vi "transfer char run_subvi_7_25_12b_JW.vi"(0 "VISA session":refnum<visa-resource-name>="GPIB0::17::INSTR", 5 "Var1 sweep settings":T4={"start"=40.0, "stop"=-40.0, "step (linear only)"=-1.0, "sweep spacing (linear: 0)"=0, "sweep mode"=FALSE, "compliance (V)"=100.0, "compliance (A)"=0.001} {"compliance (A)" format="%^.2e"; "compliance (V)" format="%.2f"; "sweep spacing (linear: 0)" items=["linear", "log 10", "log 25", "log 50"]; "step (linear only)" format="%.2f"; "stop" format="%.2f"; "start" format="%.2f"}, 7 "Var2 step settings":T3={"compliance (A)"=0.001, "compliance (V)"=100.0, "start"=-2.0, "total points"=2, "step"=-38.0} {"step" format="%.2f"; "start" format="%.2f"; "compliance (V)" format="%.2f"; "compliance (A)" format="%^.2e"}, 9 "integration time":u32(slide) scale=0.0..2.0, 11 "Input Path":path, 13 "Sample Properties:":T1 {"Date Created" format="%<%x>T"}) -> (1 "Trap Density-STS":dbl, 3 "Trap Density-VT":dbl, 4 "Mobility":dbl, 6 "graphic display":cluster{"trace":dbl[], "trace":dbl[]}(graph), 8 "On/Off Current":dbl, 10 "XY Graph":cluster{dbl[], "trace":dbl[]}[](graph), 12 "Vt":dbl, 14 "STS":dbl, 15 "error?":errorcluster)   [LabVIEW 2011]
uses:
  <vilib>/Utility/file.llb/Write To Spreadsheet File (DBL).vi
  <vilib>/Utility/file.llb/Read From Spreadsheet File (string).vi
  <vilib>/Utility/file.llb/Write To Spreadsheet File (string).vi
  <vilib>/Analysis/NI_AALPro.lvlib
panel:
  out "Test Array":string[][](array[string])
  out "Array":string[][](array[string])
  in  "Output Path":path
  in  "Temp (K)":dbl=0.001 format="%^.2e"
  in  "NumPts":dbl=5.0
  out "Numeric":dbl
  out "Max R":i32[](listbox)
  out "min r":dbl
  out "max r":dbl
  out "error? 2":errorcluster
  in  "MAXIMUM":ext format="%.2e"
  in  "MINIMUM":ext=-1e-05 format="%_2e"
  out "graphic display 2":cluster{"trace":dbl[], "trace":dbl[]}(graph)
  in  "Y1 axis":string="Id"
  in  "Y2 axis settings":T2 {"MAXIMUM" format="%.9f"; "MINIMUM" format="%.9f"}
  in  "wait time parameter":dbl=1.0
  in  "Value (Either V or A) 4":dbl
  in  "Value (Either V or A) 3":dbl
  in  "Value (Either V or A) 2":dbl
  in  "Value (V or A)":dbl
  in  "compliance (A)":dbl=0.001 format="%^.2e"
  in  "compliance (V)":dbl=100.0 format="%^.2e"
  in  "Iname":string="Is"
  in  "Vname":string="Vs"
  in  "Function":u16(ring)=4 items=["disabled", "Var1", "Var2", "Var1'", "Constant"]
  in  "Mode":u16(ring)=4 items=["V", "I", "VPulse", "IPulse", "Common"]
  in  "Iname 4":string="I4"
  in  "Vname 4":string="V4"
  in  "Function 4":u16(ring)=4 items=["disabled", "Var1", "Var2", "Var1'", "Constant"]
  in  "Mode 4":u16(ring) items=["V", "I", "VPulse", "IPulse", "Common"]
  in  "Iname 3":string="Ig"
  in  "Vname 3":string="Vg"
  in  "Function 3":u16(ring)=1 items=["disabled", "Var1", "Var2", "Var1'", "Constant"]
  in  "Mode 3":u16(ring) items=["V", "I", "VPulse", "IPulse", "Common"]
  in  "Iname 2":string="Id"
  in  "Vname 2":string="Vd"
  in  "Function 2":u16(ring)=2 items=["disabled", "Var1", "Var2", "Var1'", "Constant"]
  in  "Mode 2":u16(ring) items=["V", "I", "VPulse", "IPulse", "Common"]
  in  "reset":bool=TRUE
  # "SMU1"
  # "SMU2"
  # "SMU3"
  # "SMU4"
  # "Sample Properties:"
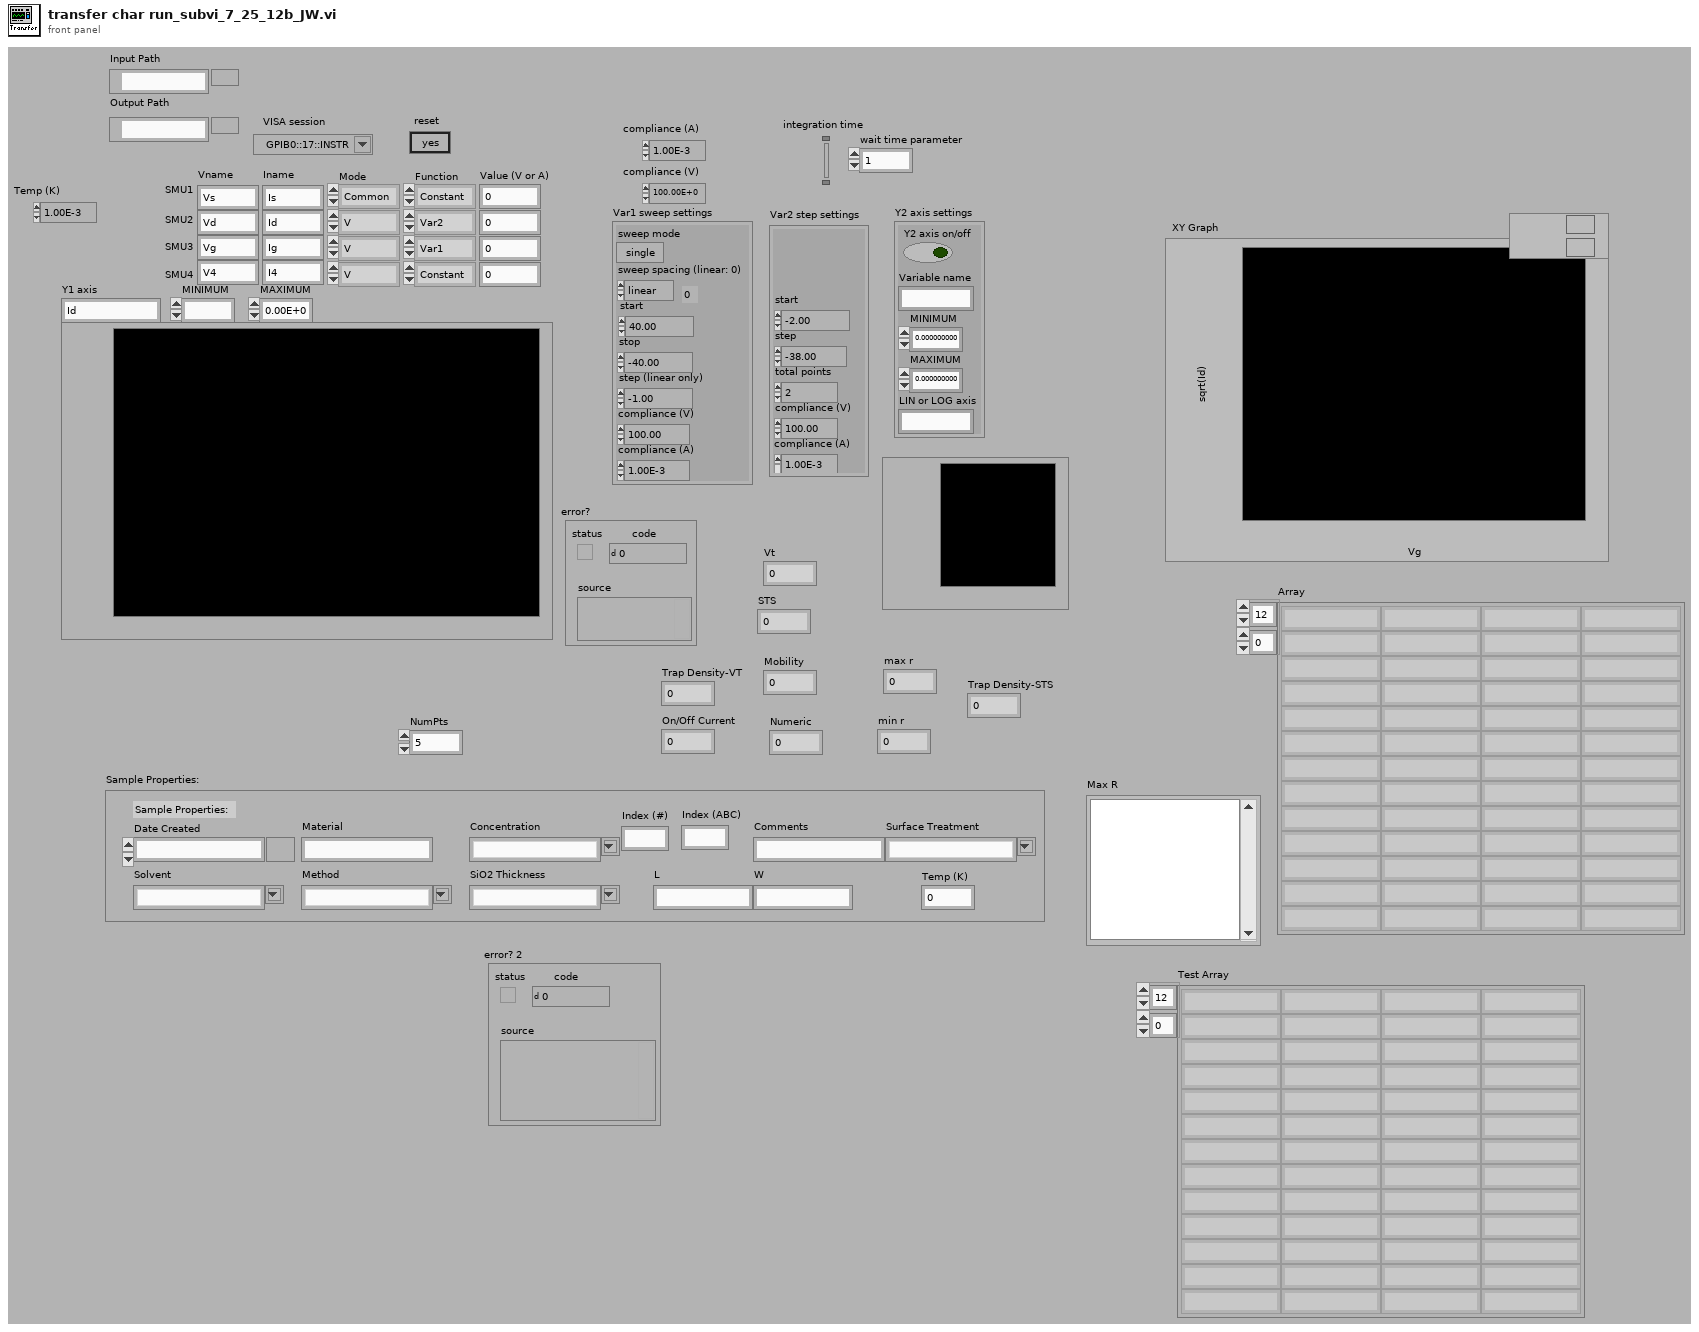
[diagram p1: front panel]
types:
  T1 = cluster{"Date Created":timestamp, "Material":string, "Solvent":string, "Concentration":string, "Method":string, "SiO2 Thickness":string, "Index (#)":string, "Index (ABC)":string, "L":string, "W":string, "Surface Treatment":string, "Comments":string, "Temp (K)":dbl}
  T2 = cluster{"Y2 axis on/off":bool, "MINIMUM":ext, "MAXIMUM":ext, "Variable name":string, "LIN or LOG axis":string}
  T3 = cluster{"compliance (A)":dbl, "compliance (V)":dbl, "start":dbl, "total points":u16, "step":dbl}
  T4 = cluster{"start":dbl, "stop":dbl, "step (linear only)":dbl, "sweep spacing (linear: 0)":u16, "sweep mode":bool, "compliance (V)":dbl, "compliance (A)":dbl}
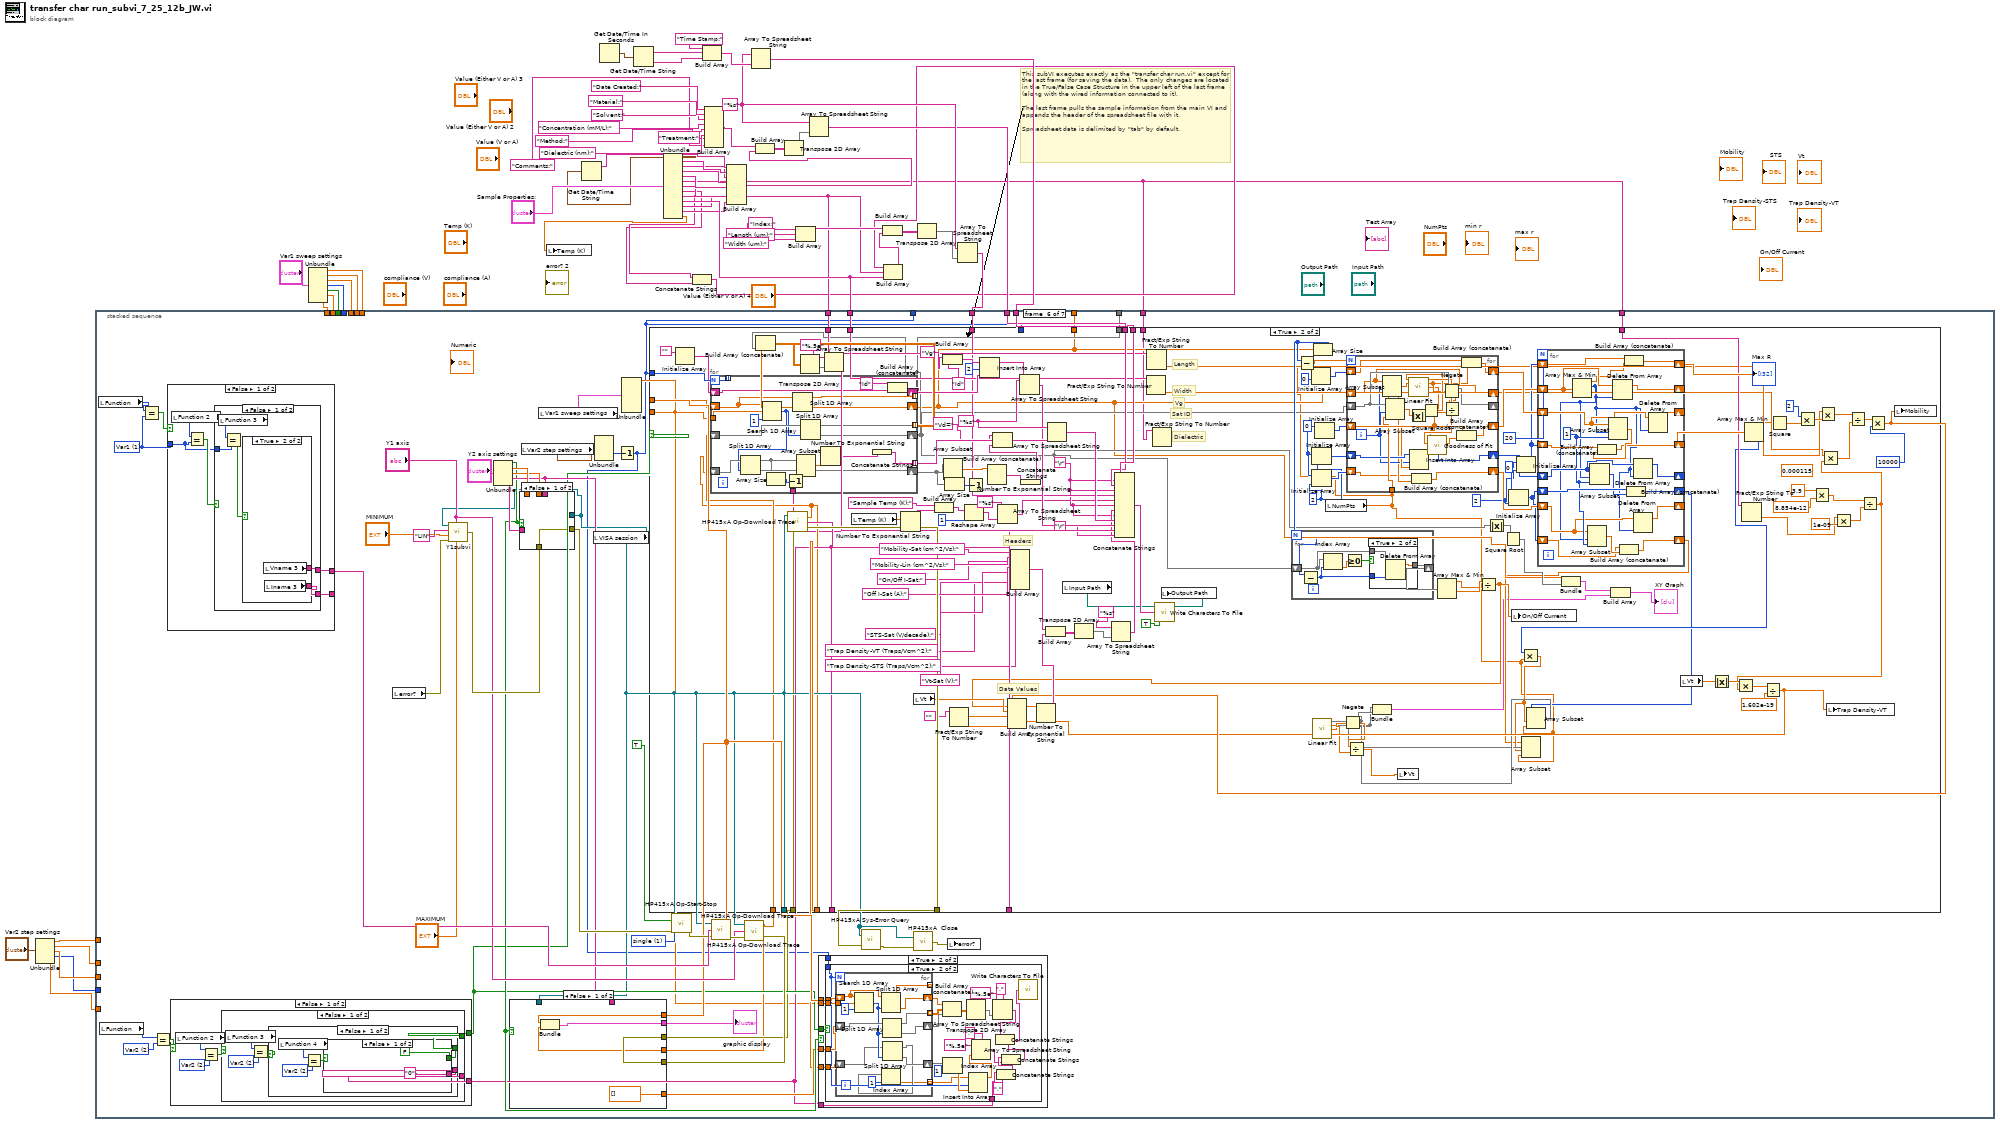
[diagram p0: block diagram]
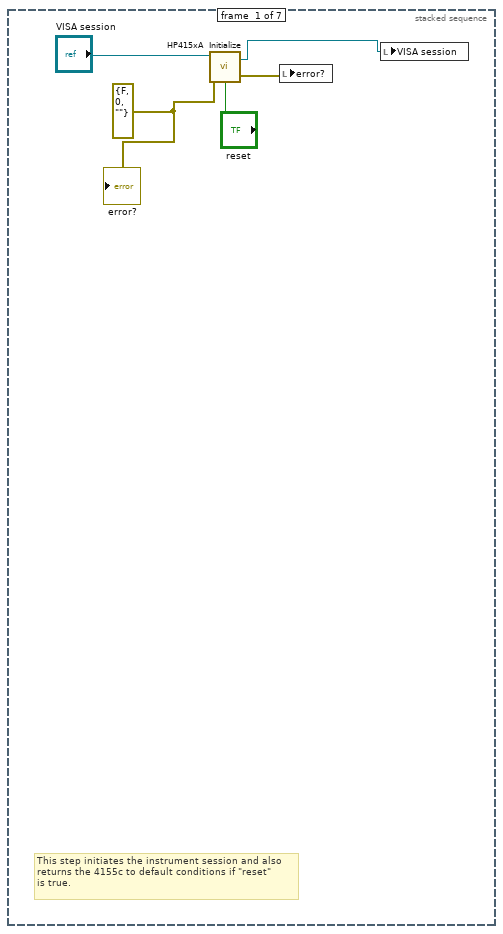
[diagram p2: hidden frame]
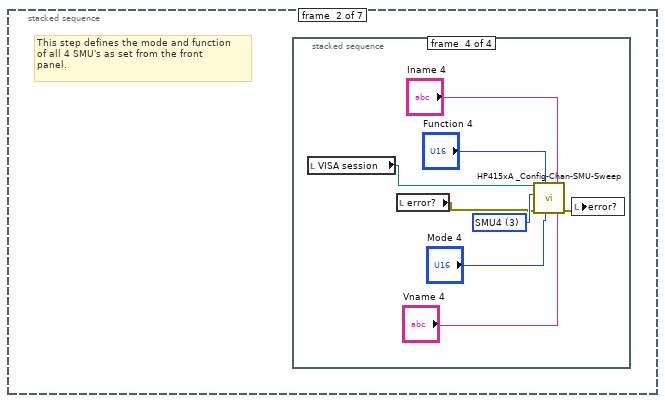
[diagram p3: hidden frame]
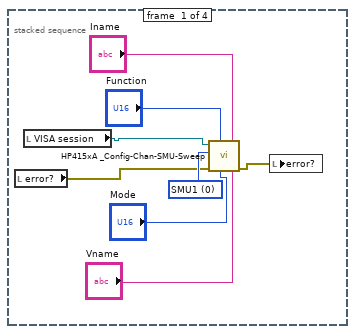
[diagram p4: hidden frame]
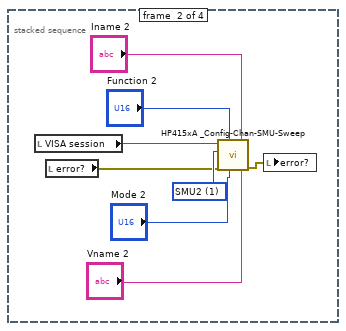
[diagram p5: hidden frame]
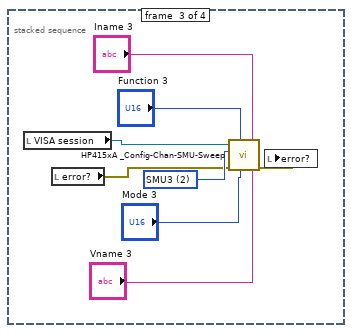
[diagram p6: hidden frame]
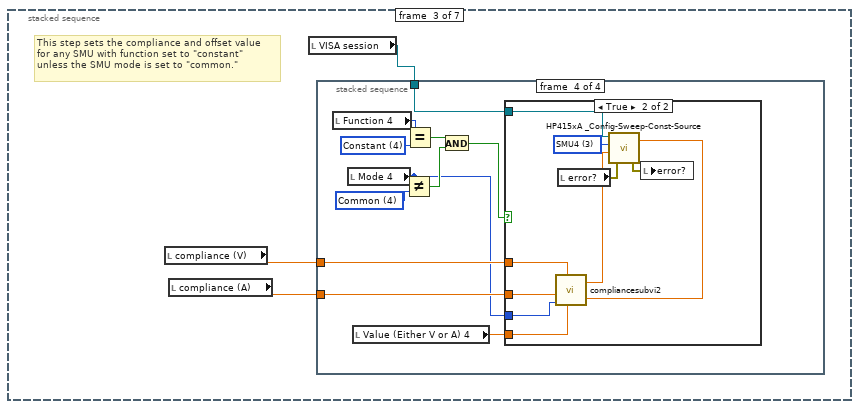
[diagram p7: hidden frame]
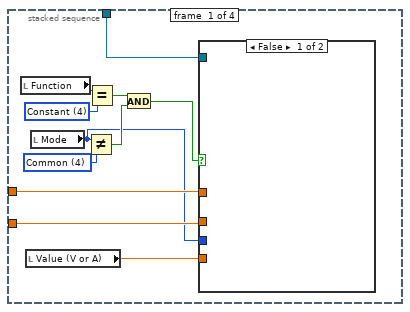
[diagram p8: hidden frame]
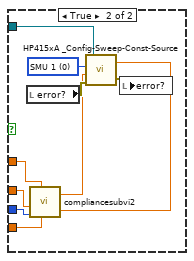
[diagram p9: hidden frame]
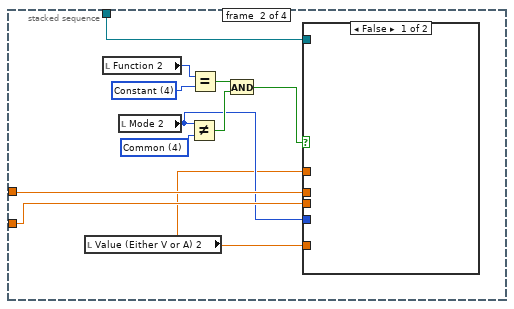
[diagram p10: hidden frame]
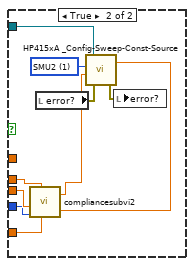
[diagram p11: hidden frame]
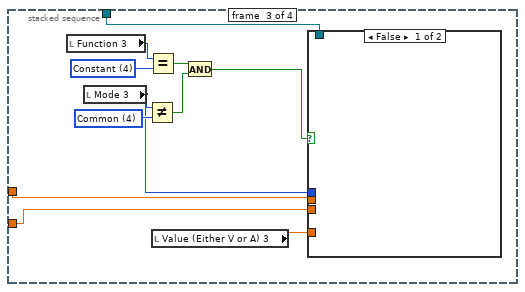
[diagram p12: hidden frame]
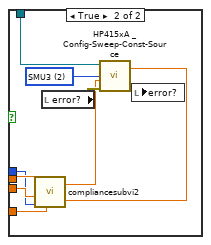
[diagram p13: hidden frame]
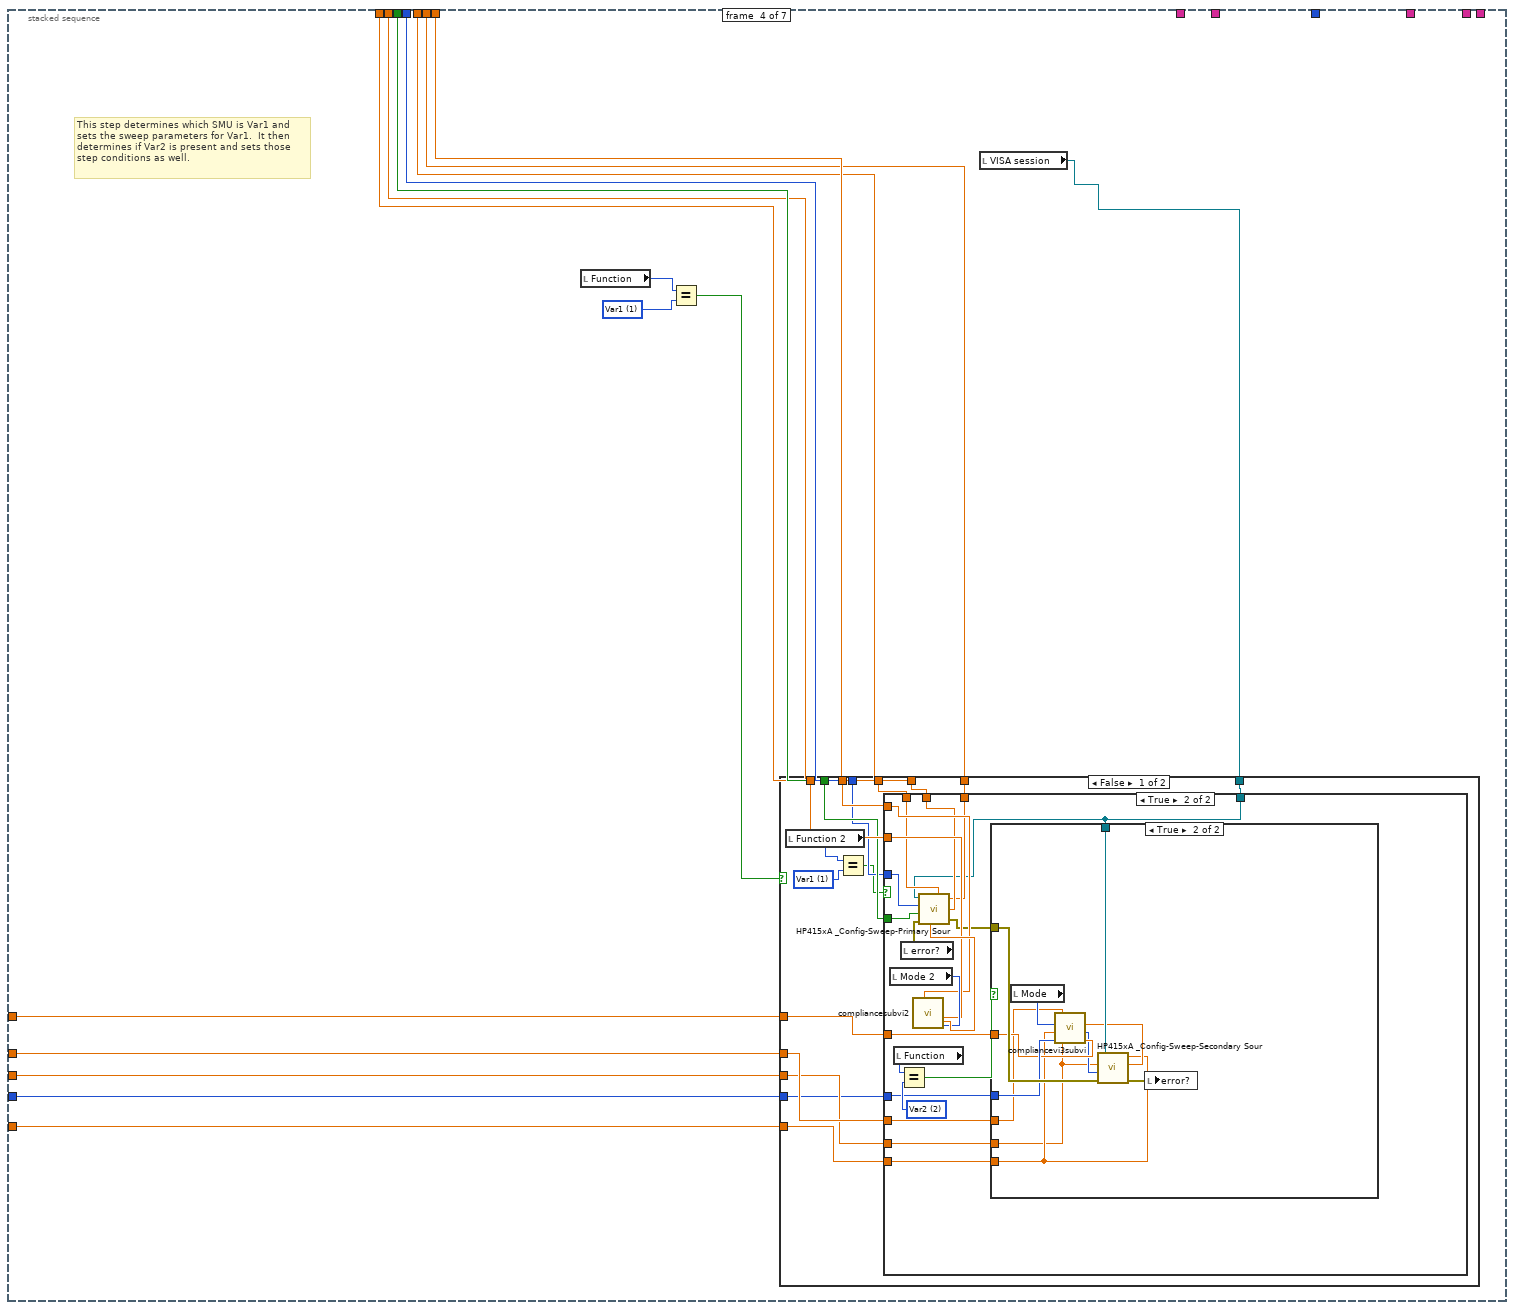
[diagram p15: hidden frame]
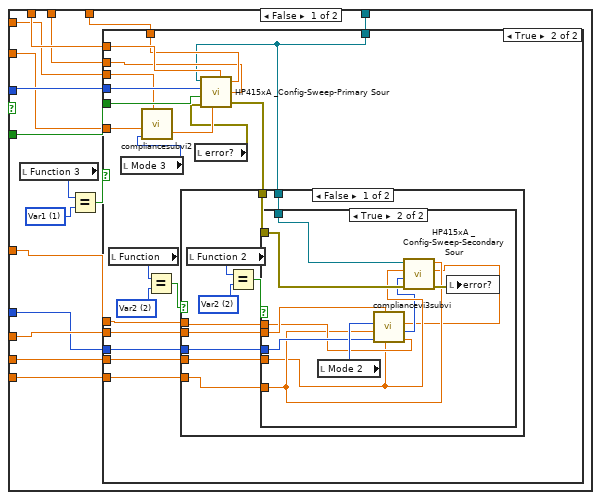
[diagram p16: hidden frame]
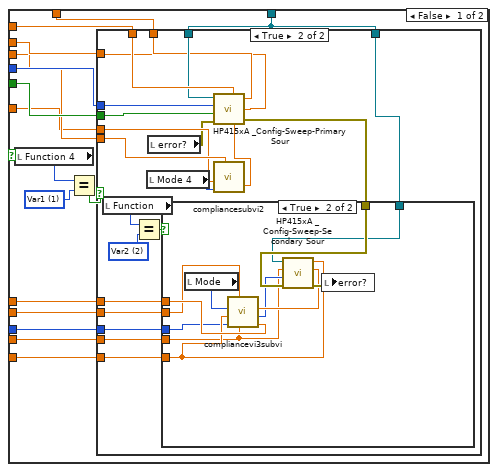
[diagram p17: hidden frame]
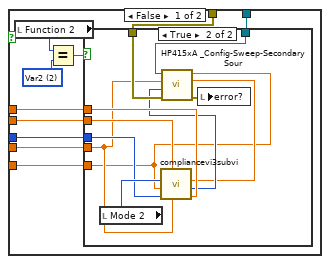
[diagram p19: hidden frame]
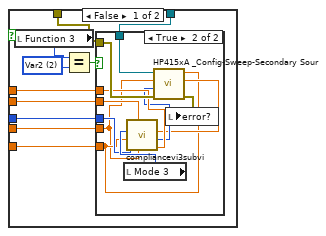
[diagram p20: hidden frame]
diagram:
  w31 = "%s"
  # "This subVI executes exactly as the \"transfer char run.vi\" except for the last frame (for saving the data).  The only changes are located in the True/False Case Structure in the upper left of the last frame (along with the wired information connected to it). \n\nThe last frame pulls the sample information from the main VI and appends the header of the spreadsheet file with it.\n\nSpreadsheet data is delimited by \"tab\" by default."
  n1 = Unbundle("Var2 step settings") -> ("compliance (A)"=w49:dbl, "compliance (V)"=w48:dbl, "start"=w47:dbl, "total points"=w46:u16, "step"=w45:dbl)
  n2 = Unbundle("Var1 sweep settings") -> ("start"=w57:dbl, "stop"=w56:dbl, "step (linear only)"=w55:dbl, "sweep spacing (linear: 0)"=w54:u16, "sweep mode"=w53:bool, "compliance (V)"=w52:dbl, "compliance (A)"=w51:dbl)
  n3 = Get Date/Time In Seconds() -> (seconds since 1Jan1904=w38:timestamp)
  n4 = Get Date/Time String(seconds (now)=w38) -> (date string=w37:string, time string=w36:string)  [unwired: 2 in]
  n5 = Unbundle("Sample Properties:") -> ("Date Created"=w16:timestamp, "Material"=w15:string, "Solvent"=w11:string, "Concentration"=w10:string, "Method"=w14:string, "SiO2 Thickness"=w1:string, "Index (#)"=w5:string, "Index (ABC)"=w4:string, "L"=w8:string, "W"=w9:string, "Surface Treatment"=w7:string, "Comments"=w6:string, "Temp (K)"=w2:dbl)
  n6 = local write "Temp (K)"(w2) -> ()
  n7 = Get Date/Time String(seconds (now)=w16) -> (date string=w43:string)  [unwired: 2 in, 1 out]
  n8 = Concatenate Strings(w5, w4) -> (w3:string)
  n9 = Build Array("Time Stamp:", w37, w36) -> (w35:string[])
  n10 = Build Array("Date Created:", "Material:", "Solvent:", "Concentration (mM/L):", "Method:", "Dielectric (nm):", "Treatment:", "Comments:") -> (w26:string[])
  n11 = Build Array(w43, w15, w11, w10, w14, w1, w7, w6) -> (w25:string[])
  n12 = Array To Spreadsheet String(array=w35, 3:w31) -> (spreadsheet string=w27:string)  [unwired: 1 in]
  n13 = Build Array(w26, w25) -> (w24:string[][])
  n14 = Transpose 2D Array(2D array=w24) -> (transposed array=w23:string[][])
  n15 = Build Array("Index:", "Length (um):", "Width (um):") -> (w22:string[])
  n16 = Array To Spreadsheet String(array=w23, 3:w31) -> (spreadsheet string=w30:string)  [unwired: 1 in]
  n17 = Build Array(w3, w8, w9) -> (w21:string[])
  n18 = Build Array(w22, w21) -> (w20:string[][])
  n19 = Transpose 2D Array(2D array=w20) -> (transposed array=w19:string[][])
  n20 = Array To Spreadsheet String(array=w19, 3:w31) -> (spreadsheet string=w18:string)  [unwired: 1 in]
  n21 = stacked-sequence {
    tunnel: w57 -> [_ _ _ w194 _ _ _]
    tunnel: w56 -> [_ _ _ w193 _ _ _]
    tunnel: w55 -> [_ _ _ w192 _ _ _]
    tunnel: w54 -> [_ _ _ w191 _ _ _]
    tunnel: w53 -> [_ _ _ w190 _ _ _]
    tunnel: w52 -> [_ _ _ w189 _ _ _]
    tunnel: w51 -> [_ _ _ w188 _ _ _]
    tunnel: w49 -> [_ _ _ w187 _ _ _]
    tunnel: w48 -> [_ _ _ w186 _ _ _]
    tunnel: w47 -> [_ _ _ w185 _ _ _]
    tunnel: w46 -> [_ _ _ w184 _ _ _]
    tunnel: w45 -> [_ _ _ w183 _ _ _]
    tunnel: w27 -> [_ _ _ _ _ w558 _]
    tunnel: w30 -> [_ _ _ _ _ w557 _]
    tunnel: w18 -> [_ _ _ _ _ w556 _]
    tunnel: [_ _ _ _ _ w555 _] -> _
    tunnel: [_ _ _ _ _ w554 _] -> _
    tunnel: [_ _ _ _ _ w551 _] -> _
    tunnel: w9 -> [_ _ _ _ _ w553 _]
    tunnel: w8 -> [_ _ _ _ _ w552 _]
    tunnel: w1 -> [_ _ _ _ _ w550 _]
    tunnel: w1 -> [_ _ _ _ _ w549 _]
    frame #0 {
      w62 = errorcluster {"status"=FALSE, "code"=0, "source"=""} ("error out")
      # "This step initiates the instrument session and also\nreturns the 4155c to default conditions if \"reset\"\nis true."
      n22 = call "HP415xA  Initialize.vi"("instrument descriptor"="VISA session", "reset"="reset", "error in (no error)"=w62) -> ("VISA session"=w59:refnum<visa-resource-name>, "error out"=w61:errorcluster)  [unwired: 2 in]
      n23 = local write "error?"(w61) -> ()
      n24 = local write "VISA session"(w59) -> ()
      "error?" <- w62
    }
    frame #1 {
      # "This step defines the mode and function\nof all 4 SMU's as set from the front\npanel."
      n25 = stacked-sequence {
        frame #0 {
          w71 = u32 0 items=["SMU1  ", "SMU2  ", "SMU3  ", "SMU4  ", "SMU5  ", "SMU6  "] ("unit to configure")
          n26 = local read "error?"() -> (w66:errorcluster)
          n27 = local read "VISA session"() -> (w64:refnum<visa-resource-name>)
          n28 = call "HP415xA _Config-Chan-SMU-Sweep.vi"("V name (max 6 chars)"="Vname", "I name (max 6 chars)"="Iname", "mode"="Mode", "function"="Function", "error in (no error)"=w66, "unit to configure"=w71, "VISA session"=w64) -> ("error out"=w65:errorcluster)  [unwired: 2 in]
          n29 = local write "error?"(w65) -> ()
        }
        frame #1 {
          w75 = u32 1 items=["SMU1  ", "SMU2  ", "SMU3  ", "SMU4  ", "SMU5  ", "SMU6  "] ("unit to configure")
          n30 = local read "VISA session"() -> (w72:refnum<visa-resource-name>)
          n31 = local read "error?"() -> (w73:errorcluster)
          n32 = call "HP415xA _Config-Chan-SMU-Sweep.vi"("V name (max 6 chars)"="Vname 2", "I name (max 6 chars)"="Iname 2", "mode"="Mode 2", "function"="Function 2", "error in (no error)"=w73, "unit to configure"=w75, "VISA session"=w72) -> ("error out"=w74:errorcluster)  [unwired: 2 in]
          n33 = local write "error?"(w74) -> ()
        }
        frame #2 {
          w83 = u32 2 items=["SMU1  ", "SMU2  ", "SMU3  ", "SMU4  ", "SMU5  ", "SMU6  "] ("unit to configure")
          n34 = local read "VISA session"() -> (w80:refnum<visa-resource-name>)
          n35 = local read "error?"() -> (w81:errorcluster)
          n36 = call "HP415xA _Config-Chan-SMU-Sweep.vi"("V name (max 6 chars)"="Vname 3", "I name (max 6 chars)"="Iname 3", "mode"="Mode 3", "function"="Function 3", "error in (no error)"=w81, "unit to configure"=w83, "VISA session"=w80) -> ("error out"=w82:errorcluster)  [unwired: 2 in]
          n37 = local write "error?"(w82) -> ()
        }
        frame #3 {
          w91 = u32 3 items=["SMU1  ", "SMU2  ", "SMU3  ", "SMU4  ", "SMU5  ", "SMU6  "] ("unit to configure")
          n38 = local read "VISA session"() -> (w88:refnum<visa-resource-name>)
          n39 = local read "error?"() -> (w90:errorcluster)
          n40 = call "HP415xA _Config-Chan-SMU-Sweep.vi"("V name (max 6 chars)"="Vname 4", "I name (max 6 chars)"="Iname 4", "mode"="Mode 4", "function"="Function 4", "error in (no error)"=w90, "unit to configure"=w91, "VISA session"=w88) -> ("error out"=w89:errorcluster)  [unwired: 2 in]
          n41 = local write "error?"(w89) -> ()
        }
      }
    }
    frame #2 {
      # "This step sets the compliance and offset value\nfor any SMU with function set to \"constant\"\nunless the SMU mode is set to \"common.\""
      n42 = local read "compliance (V)"() -> (w97:dbl)
      n43 = local read "compliance (A)"() -> (w98:dbl)
      n44 = local read "VISA session"() -> (w96:refnum<visa-resource-name>)
      n45 = stacked-sequence {
        tunnel: w96 -> [w107 w127 w146 w166]
        tunnel: w98 -> [w101 w123 w144 w164]
        tunnel: w97 -> [w100 w122 w143 w165]
        frame #0 {
          w105 = u16 4 items=["V", "I", "VPulse", "IPulse", "Common"] ("Mode")
          w109 = u16 4 items=["disabled", "Var1", "Var2", "Var1'", "Constant"] ("Function")
          n46 = local read "Function"() -> (w108:u16)
          n47 = local read "Value (V or A)"() -> (w102:dbl)
          n48 = local read "Mode"() -> (w99:u16)
          n49 = Not Equal?(x=w99, y=w105) -> (x != y?=w104:bool)
          n50 = Equal?(x=w108, y=w109) -> (x = y?=w106:bool)
          n51 = And(x=w106, y=w104) -> (x .and. y?=w103:bool)
          n52 = case shown="False" w103 {
            tunnel: w107 -> [_ w119]
            tunnel: w100 -> [_ w115]
            tunnel: w101 -> [_ w114]
            tunnel: w102 -> [_ w111]
            tunnel: w99 -> [_ w112]
            frame False {
            }
            frame True {
              w118 = u16 0 items=["SMU 1", "SMU2", "SMU3", "SMU4", "SMU5", "SMU6", "VSU1", "VSU2"] ("unit (SMU1:0)")
              n53 = local read "error?"() -> (w117:errorcluster)
              n54 = call "compliancesubvi2.vi"("Value1"=w111, "compliance (V)"=w115, "Mode"=w112, "compliance (A)"=w114) -> ("compliance"=w113:dbl, "constant"=w110:dbl)  [unwired: 2 in]
              n55 = call "HP415xA _Config-Sweep-Const-Source.vi"("compliance (SMUs only)"=w113, "error in (no error)"=w117, "source (V or A)"=w110, "unit (SMU1:0)"=w118, "VISA session"=w119) -> ("error out"=w116:errorcluster)
              n56 = local write "error?"(w116) -> ()
            }
          }
        }
        frame #1 {
          w124 = u16 4 items=["V", "I", "VPulse", "IPulse", "Common"] ("Mode 2")
          w125 = u16 4 items=["disabled", "Var1", "Var2", "Var1'", "Constant"] ("Function 2")
          n57 = local read "Value (Either V or A) 2"() -> (w120:dbl)
          n58 = local read "Function 2"() -> (w126:u16)
          n59 = local read "Mode 2"() -> (w121:u16)
          n60 = Not Equal?(x=w121, y=w124) -> (x != y?=w129:bool)
          n61 = Equal?(x=w126, y=w125) -> (x = y?=w130:bool)
          n62 = And(x=w130, y=w129) -> (x .and. y?=w128:bool)
          n63 = case shown="False" w128 {
            tunnel: w127 -> [_ w140]
            tunnel: w122 -> [_ w138]
            tunnel: w123 -> [_ w137]
            tunnel: w120 -> [_ _]
            tunnel: w121 -> [_ w133]
            tunnel: w120 -> [_ w132]
            frame False {
            }
            frame True {
              w139 = u16 1 items=["SMU 1", "SMU2", "SMU3", "SMU4", "SMU5", "SMU6", "VSU1", "VSU2"] ("unit (SMU1:0)")
              n64 = call "compliancesubvi2.vi"("Value1"=w132, "compliance (V)"=w138, "Mode"=w133, "compliance (A)"=w137) -> ("compliance"=w136:dbl, "constant"=w131:dbl)  [unwired: 2 in]
              n65 = local read "error?"() -> (w135:errorcluster)
              n66 = call "HP415xA _Config-Sweep-Const-Source.vi"("compliance (SMUs only)"=w136, "error in (no error)"=w135, "source (V or A)"=w131, "unit (SMU1:0)"=w139, "VISA session"=w140) -> ("error out"=w134:errorcluster)
              n67 = local write "error?"(w134) -> ()
            }
          }
        }
        frame #2 {
          w148 = u16 4 items=["V", "I", "VPulse", "IPulse", "Common"] ("Mode 2")
          w149 = u16 4 items=["disabled", "Var1", "Var2", "Var1'", "Constant"] ("Function 2")
          n68 = local read "Function 3"() -> (w147:u16)
          n69 = local read "Mode 3"() -> (w142:u16)
          n70 = Not Equal?(x=w142, y=w148) -> (x != y?=w150:bool)
          n71 = Equal?(x=w147, y=w149) -> (x = y?=w151:bool)
          n72 = local read "Value (Either V or A) 3"() -> (w145:dbl)
          n73 = And(x=w151, y=w150) -> (x .and. y?=w141:bool)
          n74 = case shown="False" w141 {
            tunnel: w146 -> [_ w159]
            tunnel: w145 -> [_ w153]
            tunnel: w144 -> [_ w156]
            tunnel: w143 -> [_ w155]
            tunnel: w142 -> [_ w154]
            frame False {
            }
            frame True {
              w158 = u16 2 items=["SMU 1", "SMU2", "SMU3", "SMU4", "SMU5", "SMU6", "VSU1", "VSU2"] ("unit (SMU1:0)")
              n75 = call "compliancesubvi2.vi"("Value1"=w153, "compliance (V)"=w155, "Mode"=w154, "compliance (A)"=w156) -> ("compliance"=w157:dbl, "constant"=w152:dbl)  [unwired: 2 in]
              n76 = local read "error?"() -> (w161:errorcluster)
              n77 = call "HP415xA _Config-Sweep-Const-Source.vi"("compliance (SMUs only)"=w157, "error in (no error)"=w161, "source (V or A)"=w152, "unit (SMU1:0)"=w158, "VISA session"=w159) -> ("error out"=w160:errorcluster)
              n78 = local write "error?"(w160) -> ()
            }
          }
        }
        frame #3 {
          w168 = u16 4 items=["V", "I", "VPulse", "IPulse", "Common"] ("Mode 4")
          w169 = u16 4 items=["disabled", "Var1", "Var2", "Var1'", "Constant"] ("Function 4")
          n79 = local read "Function 4"() -> (w170:u16)
          n80 = local read "Mode 4"() -> (w163:u16)
          n81 = local read "Value (Either V or A) 4"() -> (w162:dbl)
          n82 = Not Equal?(x=w163, y=w168) -> (x != y?=w171:bool)
          n83 = Equal?(x=w170, y=w169) -> (x = y?=w172:bool)
          n84 = And(x=w172, y=w171) -> (x .and. y?=w167:bool)
          n85 = case shown="True" w167 {
            tunnel: w166 -> [_ w181]
            tunnel: w165 -> [_ w177]
            tunnel: w164 -> [_ w178]
            tunnel: w163 -> [_ w176]
            tunnel: w162 -> [_ w175]
            frame False {
            }
            frame True {
              w182 = u16 3 items=["SMU 1", "SMU2", "SMU3", "SMU4", "SMU5", "SMU6", "VSU1", "VSU2"] ("unit (SMU1:0)")
              n86 = call "compliancesubvi2.vi"("Value1"=w175, "compliance (V)"=w177, "Mode"=w176, "compliance (A)"=w178) -> ("compliance"=w174:dbl, "constant"=w173:dbl)  [unwired: 2 in]
              n87 = local read "error?"() -> (w180:errorcluster)
              n88 = call "HP415xA _Config-Sweep-Const-Source.vi"("compliance (SMUs only)"=w174, "error in (no error)"=w180, "source (V or A)"=w173, "unit (SMU1:0)"=w182, "VISA session"=w181) -> ("error out"=w179:errorcluster)
              n89 = local write "error?"(w179) -> ()
            }
          }
        }
      }
    }
    frame #3 {
      w198 = u16 1 items=["disabled", "Var1", "Var2", "Var1'", "Constant"] ("Function")
      # "This step determines which SMU is Var1 and\nsets the sweep parameters for Var1.  It then\ndetermines if Var2 is present and sets those\nstep conditions as well."
      n90 = local read "Function"() -> (w197:u16)
      n91 = Equal?(x=w197, y=w198) -> (x = y?=w196:bool)
      n92 = local read "VISA session"() -> (w195:refnum<visa-resource-name>)
      n93 = case shown="False" w196 {
        tunnel: w189 -> [w211 w487]
        tunnel: w188 -> [w212 w486]
        tunnel: w191 -> [w209 w485]
        tunnel: w190 -> [w210 w484]
        tunnel: w192 -> [w206 w483]
        tunnel: w193 -> [w205 w482]
        tunnel: w194 -> [w207 w481]
        tunnel: w195 -> [w208 w470]
        tunnel: w187 -> [w203 w476]
        tunnel: w186 -> [w202 w475]
        tunnel: w185 -> [w201 w474]
        tunnel: w184 -> [w200 w473]
        tunnel: w183 -> [w199 w472]
        frame False {
          w214 = u16 1 items=["disabled", "Var1", "Var2", "Var1'", "Constant"] ("Function")
          n94 = local read "Function 2"() -> (w213:u16)
          n95 = Equal?(x=w213, y=w214) -> (x = y?=w204:bool)
          n96 = case shown="True" w204 {
            tunnel: w212 -> [w220 w413]
            tunnel: w211 -> [w221 w412]
            tunnel: w210 -> [w222 w411]
            tunnel: w209 -> [w223 w410]
            tunnel: w208 -> [w227 w399]
            tunnel: w207 -> [w226 w409]
            tunnel: w206 -> [w224 w408]
            tunnel: w205 -> [w225 w407]
            tunnel: w203 -> [w219 w402]
            tunnel: w202 -> [w218 w401]
            tunnel: w201 -> [w216 w400]
            tunnel: w200 -> [w217 w397]
            tunnel: w199 -> [w215 w396]
            frame False {
              w230 = u16 1 items=["disabled", "Var1", "Var2", "Var1'", "Constant"] ("Function")
              n97 = local read "Function 3"() -> (w229:u16)
              n98 = Equal?(x=w229, y=w230) -> (x = y?=w228:bool)
              n99 = case shown="True" w228 {
                tunnel: w227 -> [w231 w324]
                tunnel: w226 -> [w243 w341]
                tunnel: w225 -> [w240 w340]
                tunnel: w224 -> [w239 w339]
                tunnel: w223 -> [w242 w338]
                tunnel: w222 -> [w241 w337]
                tunnel: w221 -> [w238 w336]
                tunnel: w220 -> [w237 w335]
                tunnel: w219 -> [w236 w328]
                tunnel: w218 -> [w235 w327]
                tunnel: w217 -> [w234 w326]
                tunnel: w216 -> [w233 w323]
                tunnel: w215 -> [w232 w322]
                frame False {
                  w246 = u16 1 items=["disabled", "Var1", "Var2", "Var1'", "Constant"] ("Function")
                  n100 = local read "Function 4"() -> (w245:u16)
                  n101 = Equal?(x=w245, y=w246) -> (x = y?=w244:bool)
                  n102 = case shown="True" w244 {
                    tunnel: w243 -> [_ w265]
                    tunnel: w231 -> [_ w264]
                    tunnel: w242 -> [_ w263]
                    tunnel: w241 -> [_ w262]
                    tunnel: w240 -> [_ w261]
                    tunnel: w239 -> [_ w260]
                    tunnel: w238 -> [_ w259]
                    tunnel: w237 -> [_ w258]
                    tunnel: w236 -> [_ w253]
                    tunnel: w235 -> [_ w252]
                    tunnel: w234 -> [_ w251]
                    tunnel: w233 -> [_ w250]
                    tunnel: w232 -> [_ w249]
                    tunnel: w231 -> [_ w247]
                    frame False {
                    }
                    frame True {
                      w256 = u16 2 items=["disabled", "Var1", "Var2", "Var1'", "Constant"] ("Function")
                      n103 = local read "Function"() -> (w255:u16)
                      n104 = Equal?(x=w255, y=w256) -> (x = y?=w254:bool)
                      n105 = local read "Mode 4"() -> (w267:u16)
                      n106 = local read "error?"() -> (w257:errorcluster)
                      n107 = call "compliancesubvi2.vi"("compliance (V)"=w259, "Mode"=w267, "compliance (A)"=w258) -> ("compliance"=w266:dbl)  [unwired: 3 in, 1 out]
                      n108 = call "HP415xA _Config-Sweep-Primary Sour.vi"("step (linear only)"=w260, "stop"=w261, "start"=w265, "compliance"=w266, "error in (no error)"=w257, "sweep mode"=w262, "sweep spacing (linear: 0)"=w263, "VISA session"=w264) -> ("error out"=w248:errorcluster)  [unwired: 2 in]
                      n109 = case shown="True" w254 {
                        tunnel: w253 -> [w274 w317]
                        tunnel: w252 -> [w273 w312]
                        tunnel: w251 -> [w272 w311]
                        tunnel: w250 -> [w271 w313]
                        tunnel: w249 -> [w270 w316]
                        tunnel: w248 -> [w269 w319]
                        tunnel: w247 -> [w268 w318]
                        frame False {
                          w277 = u16 2 items=["disabled", "Var1", "Var2", "Var1'", "Constant"] ("Function")
                          n110 = local read "Function 2"() -> (w276:u16)
                          n111 = Equal?(x=w276, y=w277) -> (x = y?=w275:bool)
                          n112 = case shown="True" w275 {
                            tunnel: w274 -> [w285 w305]
                            tunnel: w273 -> [w284 w306]
                            tunnel: w272 -> [w283 w304]
                            tunnel: w271 -> [w282 w302]
                            tunnel: w270 -> [w281 w300]
                            tunnel: w269 -> [w280 w310]
                            tunnel: w268 -> [w278 w309]
                            frame False {
                              w287 = u16 2 items=["disabled", "Var1", "Var2", "Var1'", "Constant"] ("Function")
                              n113 = local read "Function 3"() -> (w279:u16)
                              n114 = Equal?(x=w279, y=w287) -> (x = y?=w286:bool)
                              n115 = case shown="True" w286 {
                                tunnel: w285 -> [_ w293]
                                tunnel: w284 -> [_ w294]
                                tunnel: w283 -> [_ w295]
                                tunnel: w282 -> [_ w289]
                                tunnel: w281 -> [_ w290]
                                tunnel: w280 -> [w288 w299]
                                tunnel: w278 -> [_ w298]
                                frame False {
                                n116 = local write "error?"(w288) -> ()
                                }
                                frame True {
                                n117 = local read "Mode 3"() -> (w297:u16)
                                n118 = call "compliancevi3subvi.vi"("compliance (A)"=w293, "start"=w289, "compliance (V)"=w294, "total points"=w295, "step"=w290, "Mode"=w297) -> ("total points 2"=w292:u16, "compliance"=w291:dbl)  [unwired: 1 in, 1 out]
                                n119 = call "HP415xA _Config-Sweep-Secondary Sour.vi"("compliance"=w291, "step"=w290, "error in (no error)"=w299, "total points"=w292, "start"=w289, "VISA session"=w298) -> ("error out"=w296:errorcluster)  [unwired: 1 in]
                                n120 = local write "error?"(w296) -> ()
                                }
                              }
                            }
                            frame True {
                              n121 = local read "Mode 2"() -> (w308:u16)
                              n122 = call "compliancevi3subvi.vi"("compliance (A)"=w305, "start"=w302, "compliance (V)"=w306, "total points"=w304, "step"=w300, "Mode"=w308) -> ("total points 2"=w303:u16, "compliance"=w301:dbl)  [unwired: 1 in, 1 out]
                              n123 = call "HP415xA _Config-Sweep-Secondary Sour.vi"("compliance"=w301, "step"=w300, "error in (no error)"=w310, "total points"=w303, "start"=w302, "VISA session"=w309) -> ("error out"=w307:errorcluster)  [unwired: 1 in]
                              n124 = local write "error?"(w307) -> ()
                            }
                          }
                        }
                        frame True {
                          n125 = local read "Mode"() -> (w321:u16)
                          n126 = call "compliancevi3subvi.vi"("compliance (A)"=w317, "start"=w313, "compliance (V)"=w312, "total points"=w311, "step"=w316, "Mode"=w321) -> ("total points 2"=w314:u16, "compliance"=w315:dbl)  [unwired: 1 in, 1 out]
                          n127 = call "HP415xA _Config-Sweep-Secondary Sour.vi"("compliance"=w315, "step"=w316, "error in (no error)"=w319, "total points"=w314, "start"=w313, "VISA session"=w318) -> ("error out"=w320:errorcluster)  [unwired: 1 in]
                          n128 = local write "error?"(w320) -> ()
                        }
                      }
                    }
                  }
                }
                frame True {
                  w331 = u16 2 items=["disabled", "Var1", "Var2", "Var1'", "Constant"] ("Function")
                  n129 = local read "Function"() -> (w330:u16)
                  n130 = local read "Mode 3"() -> (w333:u16)
                  n131 = call "compliancesubvi2.vi"("compliance (V)"=w336, "Mode"=w333, "compliance (A)"=w335) -> ("compliance"=w334:dbl)  [unwired: 3 in, 1 out]
                  n132 = Equal?(x=w330, y=w331) -> (x = y?=w329:bool)
                  n133 = local read "error?"() -> (w332:errorcluster)
                  n134 = call "HP415xA _Config-Sweep-Primary Sour.vi"("step (linear only)"=w339, "stop"=w340, "start"=w341, "compliance"=w334, "error in (no error)"=w332, "sweep mode"=w337, "sweep spacing (linear: 0)"=w338, "VISA session"=w324) -> ("error out"=w325:errorcluster)  [unwired: 2 in]
                  n135 = case shown="False" w329 {
                    tunnel: w328 -> [w346 w391]
                    tunnel: w327 -> [w345 w390]
                    tunnel: w326 -> [w343 w389]
                    tunnel: w325 -> [w348 w394]
                    tunnel: w324 -> [w347 w393]
                    tunnel: w323 -> [w342 w386]
                    tunnel: w322 -> [w344 w385]
                    frame False {
                      w351 = u16 2 items=["disabled", "Var1", "Var2", "Var1'", "Constant"] ("Function")
                      n136 = local read "Function 2"() -> (w350:u16)
                      n137 = Equal?(x=w350, y=w351) -> (x = y?=w349:bool)
                      n138 = case shown="True" w349 {
                        tunnel: w348 -> [w358 w383]
                        tunnel: w347 -> [w357 w382]
                        tunnel: w346 -> [w356 w378]
                        tunnel: w345 -> [w355 w379]
                        tunnel: w344 -> [w352 w377]
                        tunnel: w343 -> [w354 w380]
                        tunnel: w342 -> [w353 w376]
                        frame False {
                          w361 = u16 2 items=["disabled", "Var1", "Var2", "Var1'", "Constant"] ("Function")
                          n139 = local read "Function 4"() -> (w360:u16)
                          n140 = Equal?(x=w360, y=w361) -> (x = y?=w359:bool)
                          n141 = case shown="True" w359 {
                            tunnel: w358 -> [w362 w371]
                            tunnel: w357 -> [_ w372]
                            tunnel: w356 -> [_ w368]
                            tunnel: w355 -> [_ w369]
                            tunnel: w354 -> [_ w367]
                            tunnel: w353 -> [_ w364]
                            tunnel: w352 -> [_ w363]
                            frame False {
                              n142 = local write "error?"(w362) -> ()
                            }
                            frame True {
                              n143 = local read "Mode 4"() -> (w373:u16)
                              n144 = call "compliancevi3subvi.vi"("compliance (A)"=w368, "start"=w364, "compliance (V)"=w369, "total points"=w367, "step"=w363, "Mode"=w373) -> ("total points 2"=w366:u16, "compliance"=w365:dbl)  [unwired: 1 in, 1 out]
                              n145 = call "HP415xA _Config-Sweep-Secondary Sour.vi"("compliance"=w365, "step"=w363, "error in (no error)"=w371, "total points"=w366, "start"=w364, "VISA session"=w372) -> ("error out"=w370:errorcluster)  [unwired: 1 in]
                              n146 = local write "error?"(w370) -> ()
                            }
                          }
                        }
                        frame True {
                          n147 = local read "Mode 2"() -> (w384:u16)
                          n148 = call "compliancevi3subvi.vi"("compliance (A)"=w378, "start"=w376, "compliance (V)"=w379, "total points"=w380, "step"=w377, "Mode"=w384) -> ("total points 2"=w375:u16, "compliance"=w374:dbl)  [unwired: 1 in, 1 out]
                          n149 = call "HP415xA _Config-Sweep-Secondary Sour.vi"("compliance"=w374, "step"=w377, "error in (no error)"=w383, "total points"=w375, "start"=w376, "VISA session"=w382) -> ("error out"=w381:errorcluster)  [unwired: 1 in]
                          n150 = local write "error?"(w381) -> ()
                        }
                      }
                    }
                    frame True {
                      n151 = local read "Mode"() -> (w395:u16)
                      n152 = call "compliancevi3subvi.vi"("compliance (A)"=w391, "start"=w386, "compliance (V)"=w390, "total points"=w389, "step"=w385, "Mode"=w395) -> ("total points 2"=w388:u16, "compliance"=w387:dbl)  [unwired: 1 in, 1 out]
                      n153 = call "HP415xA _Config-Sweep-Secondary Sour.vi"("compliance"=w387, "step"=w385, "error in (no error)"=w394, "total points"=w388, "start"=w386, "VISA session"=w393) -> ("error out"=w392:errorcluster)  [unwired: 1 in]
                      n154 = local write "error?"(w392) -> ()
                    }
                  }
                }
              }
            }
            frame True {
              w405 = u16 2 items=["disabled", "Var1", "Var2", "Var1'", "Constant"] ("Function")
              n155 = local read "Mode 2"() -> (w414:u16)
              n156 = local read "Function"() -> (w404:u16)
              n157 = Equal?(x=w404, y=w405) -> (x = y?=w403:bool)
              n158 = local read "error?"() -> (w406:errorcluster)
              n159 = call "compliancesubvi2.vi"("compliance (V)"=w412, "Mode"=w414, "compliance (A)"=w413) -> ("compliance"=w415:dbl)  [unwired: 3 in, 1 out]
              n160 = call "HP415xA _Config-Sweep-Primary Sour.vi"("step (linear only)"=w408, "stop"=w407, "start"=w409, "compliance"=w415, "error in (no error)"=w406, "sweep mode"=w411, "sweep spacing (linear: 0)"=w410, "VISA session"=w399) -> ("error out"=w398:errorcluster)  [unwired: 2 in]
              n161 = case shown="True" w403 {
                tunnel: w402 -> [w421 w464]
                tunnel: w401 -> [w420 w463]
                tunnel: w400 -> [w418 w459]
                tunnel: w399 -> [w423 w469]
                tunnel: w398 -> [w417 w468]
                tunnel: w397 -> [w419 w465]
                tunnel: w396 -> [w416 w461]
                frame False {
                  w425 = u16 2 items=["disabled", "Var1", "Var2", "Var1'", "Constant"] ("Function")
                  n162 = local read "Function 3"() -> (w424:u16)
                  n163 = Equal?(x=w424, y=w425) -> (x = y?=w422:bool)
                  n164 = case shown="True" w422 {
                    tunnel: w423 -> [w431 w457]
                    tunnel: w421 -> [w430 w454]
                    tunnel: w420 -> [w428 w452]
                    tunnel: w419 -> [w429 w453]
                    tunnel: w418 -> [w426 w450]
                    tunnel: w417 -> [w432 w456]
                    tunnel: w416 -> [w427 w448]
                    frame False {
                      w435 = u16 2 items=["disabled", "Var1", "Var2", "Var1'", "Constant"] ("Function")
                      n165 = local read "Function 4"() -> (w434:u16)
                      n166 = Equal?(x=w434, y=w435) -> (x = y?=w433:bool)
                      n167 = case shown="True" w433 {
                        tunnel: w432 -> [w436 w447]
                        tunnel: w431 -> [_ w446]
                        tunnel: w430 -> [_ w443]
                        tunnel: w429 -> [_ w444]
                        tunnel: w428 -> [_ w442]
                        tunnel: w427 -> [_ w438]
                        tunnel: w426 -> [_ w439]
                        frame False {
                          n168 = local write "error?"(w436) -> ()
                        }
                        frame True {
                          n169 = local read "Mode 4"() -> (w441:u16)
                          n170 = call "compliancevi3subvi.vi"("compliance (A)"=w443, "start"=w439, "compliance (V)"=w442, "total points"=w444, "step"=w438, "Mode"=w441) -> ("total points 2"=w440:u16, "compliance"=w437:dbl)  [unwired: 1 in, 1 out]
                          n171 = call "HP415xA _Config-Sweep-Secondary Sour.vi"("compliance"=w437, "step"=w438, "error in (no error)"=w447, "total points"=w440, "start"=w439, "VISA session"=w446) -> ("error out"=w445:errorcluster)  [unwired: 1 in]
                          n172 = local write "error?"(w445) -> ()
                        }
                      }
                    }
                    frame True {
                      n173 = local read "Mode 3"() -> (w458:u16)
                      n174 = call "compliancevi3subvi.vi"("compliance (A)"=w454, "start"=w450, "compliance (V)"=w452, "total points"=w453, "step"=w448, "Mode"=w458) -> ("total points 2"=w451:u16, "compliance"=w449:dbl)  [unwired: 1 in, 1 out]
                      n175 = call "HP415xA _Config-Sweep-Secondary Sour.vi"("compliance"=w449, "step"=w448, "error in (no error)"=w456, "total points"=w451, "start"=w450, "VISA session"=w457) -> ("error out"=w455:errorcluster)  [unwired: 1 in]
                      n176 = local write "error?"(w455) -> ()
                    }
                  }
                }
                frame True {
                  n177 = local read "Mode"() -> (w466:u16)
                  n178 = call "compliancevi3subvi.vi"("compliance (A)"=w464, "start"=w459, "compliance (V)"=w463, "total points"=w465, "step"=w461, "Mode"=w466) -> ("total points 2"=w460:u16, "compliance"=w462:dbl)  [unwired: 1 in, 1 out]
                  n179 = call "HP415xA _Config-Sweep-Secondary Sour.vi"("compliance"=w462, "step"=w461, "error in (no error)"=w468, "total points"=w460, "start"=w459, "VISA session"=w469) -> ("error out"=w467:errorcluster)  [unwired: 1 in]
                  n180 = local write "error?"(w467) -> ()
                }
              }
            }
          }
        }
        frame True {
          w478 = u16 2 items=["disabled", "Var1", "Var2", "Var1'", "Constant"] ("Function 2")
          n181 = local read "error?"() -> (w480:errorcluster)
          n182 = local read "Mode"() -> (w488:u16)
          n183 = local read "Function 2"() -> (w479:u16)
          n184 = call "compliancesubvi2.vi"("compliance (V)"=w487, "Mode"=w488, "compliance (A)"=w486) -> ("compliance"=w489:dbl)  [unwired: 3 in, 1 out]
          n185 = call "HP415xA _Config-Sweep-Primary Sour.vi"("step (linear only)"=w483, "stop"=w482, "start"=w481, "compliance"=w489, "error in (no error)"=w480, "sweep mode"=w484, "sweep spacing (linear: 0)"=w485, "VISA session"=w470) -> ("error out"=w471:errorcluster)  [unwired: 2 in]
          n186 = Equal?(x=w479, y=w478) -> (x = y?=w477:bool)
          n187 = case shown="True" w477 {
            tunnel: w476 -> [w495 w539]
            tunnel: w475 -> [w496 w538]
            tunnel: w474 -> [w493 w535]
            tunnel: w473 -> [w494 w537]
            tunnel: w472 -> [w492 w533]
            tunnel: w471 -> [w491 w542]
            tunnel: w470 -> [w490 w540]
            frame False {
              w499 = u16 2 items=["disabled", "Var1", "Var2", "Var1'", "Constant"] ("Function 2")
              n188 = local read "Function 3"() -> (w498:u16)
              n189 = Equal?(x=w498, y=w499) -> (x = y?=w497:bool)
              n190 = case shown="True" w497 {
                tunnel: w496 -> [w504 w522]
                tunnel: w495 -> [w505 w523]
                tunnel: w494 -> [w502 w528]
                tunnel: w493 -> [w503 w525]
                tunnel: w492 -> [w501 w524]
                tunnel: w491 -> [w506 w531]
                tunnel: w490 -> [w500 w529]
                frame False {
                  w509 = u16 2 items=["disabled", "Var1", "Var2", "Var1'", "Constant"] ("Function 2")
                  n191 = local read "Function 4"() -> (w508:u16)
                  n192 = Equal?(x=w508, y=w509) -> (x = y?=w507:bool)
                  n193 = case shown="True" w507 {
                    tunnel: w506 -> [w510 w521]
                    tunnel: w505 -> [_ w511]
                    tunnel: w504 -> [_ w512]
                    tunnel: w503 -> [_ w513]
                    tunnel: w502 -> [_ w518]
                    tunnel: w501 -> [_ w515]
                    tunnel: w500 -> [_ w519]
                    frame False {
                      n194 = local write "error?"(w510) -> ()
                    }
                    frame True {
                      n195 = local read "Mode 4"() -> (w517:u16)
                      n196 = call "compliancevi3subvi.vi"("compliance (A)"=w511, "start"=w513, "compliance (V)"=w512, "total points"=w518, "step"=w515, "Mode"=w517) -> ("total points 2"=w514:u16, "compliance"=w516:dbl)  [unwired: 1 in, 1 out]
                      n197 = call "HP415xA _Config-Sweep-Secondary Sour.vi"("compliance"=w516, "step"=w515, "error in (no error)"=w521, "total points"=w514, "start"=w513, "VISA session"=w519) -> ("error out"=w520:errorcluster)  [unwired: 1 in]
                      n198 = local write "error?"(w520) -> ()
                    }
                  }
                }
                frame True {
                  n199 = local read "Mode 3"() -> (w532:u16)
                  n200 = call "compliancevi3subvi.vi"("compliance (A)"=w523, "start"=w525, "compliance (V)"=w522, "total points"=w528, "step"=w524, "Mode"=w532) -> ("total points 2"=w527:u16, "compliance"=w526:dbl)  [unwired: 1 in, 1 out]
                  n201 = call "HP415xA _Config-Sweep-Secondary Sour.vi"("compliance"=w526, "step"=w524, "error in (no error)"=w531, "total points"=w527, "start"=w525, "VISA session"=w529) -> ("error out"=w530:errorcluster)  [unwired: 1 in]
                  n202 = local write "error?"(w530) -> ()
                }
              }
            }
            frame True {
              n203 = local read "Mode 2"() -> (w543:u16)
              n204 = call "compliancevi3subvi.vi"("compliance (A)"=w539, "start"=w535, "compliance (V)"=w538, "total points"=w537, "step"=w533, "Mode"=w543) -> ("total points 2"=w536:u16, "compliance"=w534:dbl)  [unwired: 1 in, 1 out]
              n205 = call "HP415xA _Config-Sweep-Secondary Sour.vi"("compliance"=w534, "step"=w533, "error in (no error)"=w542, "total points"=w536, "start"=w535, "VISA session"=w540) -> ("error out"=w541:errorcluster)  [unwired: 1 in]
              n206 = local write "error?"(w541) -> ()
            }
          }
        }
      }
    }
    frame #4 {
      # "This step sets the integration time."
      n207 = local read "VISA session"() -> (w544:refnum<visa-resource-name>)
      n208 = local read "error?"() -> (w548:errorcluster)
      n209 = call "HP415xA _Config-Meas-Timing.vi"("error in (no error)"=w548, "wait time parameter"="wait time parameter", "integration time"="integration time", "VISA session"=w544) -> ("error out"=w547:errorcluster)  [unwired: 2 in]
      n210 = local write "error?"(w547) -> ()
    }
    frame #5 {
      w585 = u32 1 items=["stop  ", "single  ", "single-append  ", "stress start  ", "continuous  ", "standby on  ", "standby off  ", "zero  "] ("function (stop:0)")
      w589 = u16 2 items=["disabled", "Var1", "Var2", "Var1'", "Constant"] ("Function")
      w594 = u16 1 items=["disabled", "Var1", "Var2", "Var1'", "Constant"] ("Function")
      n211 = local read "Function"() -> (w596:u16)
      n212 = local read "Function"() -> (w588:u16)
      n213 = Equal?(x=w596, y=w594) -> (x = y?=w595:bool)
      n214 = Equal?(x=w588, y=w589) -> (x = y?=w587:bool)
      n215 = case shown="False" w595 {
        tunnel: [w959 w974] -> w590
        tunnel: [w960 w973] -> _
        tunnel: w594 -> [w957 _]
        frame False {
          n216 = local read "Function 2"() -> (w961:u16)
          n217 = Equal?(x=w961, y=w957) -> (x = y?=w958:bool)
          n218 = case shown="False" w958 {
            tunnel: [w962 w972] -> w960
            tunnel: [w963 w971] -> w959
            tunnel: w957 -> [w966 _]
            frame False {
              n219 = local read "Function 3"() -> (w965:u16)
              n220 = Equal?(x=w965, y=w966) -> (x = y?=w964:bool)
              n221 = case shown="True" w964 {
                tunnel: [w968 w970] -> w963
                tunnel: [w967 w969] -> w962
                frame False {
                  n222 = local read "Vname 4"() -> (w968:string)
                  n223 = local read "Iname 4"() -> (w967:string)
                }
                frame True {
                  n224 = local read "Vname 3"() -> (w970:string)
                  n225 = local read "Iname 3"() -> (w969:string)
                }
              }
            }
            frame True {
              n226 = local read "Vname 2"() -> (w971:string)
              n227 = local read "Iname 2"() -> (w972:string)
            }
          }
        }
        frame True {
          n228 = local read "Vname"() -> (w974:string)
          n229 = local read "Iname"() -> (w973:string)
        }
      }
      n230 = case shown="False" w587 {
        tunnel: [w901 w954] -> w560
        tunnel: [w900 TRUE ("x = y?")] -> w566
        frame False {
          w904 = u16 2 items=["disabled", "Var1", "Var2", "Var1'", "Constant"] ("Function")
          n231 = local read "Function 2"() -> (w903:u16)
          n232 = Equal?(x=w903, y=w904) -> (x = y?=w902:bool)
          n233 = case shown="False" w902 {
            tunnel: [w906 w944] -> w901
            tunnel: [w905 TRUE ("x = y?")] -> w900
            frame False {
              w909 = u16 2 items=["disabled", "Var1", "Var2", "Var1'", "Constant"] ("Function")
              n234 = local read "Function 3"() -> (w908:u16)
              n235 = Equal?(x=w908, y=w909) -> (x = y?=w907:bool)
              n236 = case shown="False" w907 {
                tunnel: [w914 w934] -> w906
                tunnel: [w910 TRUE ("x = y?")] -> w905
                frame False {
                  w913 = u16 2 items=["disabled", "Var1", "Var2", "Var1'", "Constant"] ("Function")
                  n237 = local read "Function 4"() -> (w912:u16)
                  n238 = Equal?(x=w912, y=w913) -> (x = y?=w911:bool)
                  n239 = case shown="False" w911 {
                    tunnel: ["0" ("Vname 4") w924] -> w914
                    tunnel: [FALSE ("x = y?") TRUE ("x = y?")] -> w910
                    frame False {
                    }
                    frame True {
                      w918 = u16 2 items=["V", "I", "VPulse", "IPulse", "Common"] ("Mode 2")
                      w921 = u16 0 items=["V", "I", "VPulse", "IPulse", "Common"] ("Mode 2")
                      n240 = local read "Mode 4"() -> (w920:u16)
                      n241 = Equal?(x=w921, y=w920) -> (x = y?=w922:bool)
                      n242 = Equal?(x=w920, y=w918) -> (x = y?=w919:bool)
                      n243 = Or(x=w922, y=w919) -> (x .or. y?=w917:bool)
                      n244 = case shown="False" w917 {
                        tunnel: [w925 w926] -> w924
                        frame False {
                          n245 = local read "Iname 4"() -> (w925:string)
                        }
                        frame True {
                          n246 = local read "Vname 4"() -> (w926:string)
                        }
                      }
                    }
                  }
                }
                frame True {
                  w930 = u16 2 items=["V", "I", "VPulse", "IPulse", "Common"] ("Mode 2")
                  w929 = u16 0 items=["V", "I", "VPulse", "IPulse", "Common"] ("Mode 2")
                  n247 = local read "Mode 3"() -> (w928:u16)
                  n248 = Equal?(x=w929, y=w928) -> (x = y?=w932:bool)
                  n249 = Equal?(x=w928, y=w930) -> (x = y?=w931:bool)
                  n250 = Or(x=w932, y=w931) -> (x .or. y?=w927:bool)
                  n251 = case shown="False" w927 {
                    tunnel: [w935 w936] -> w934
                    frame False {
                      n252 = local read "Iname 3"() -> (w935:string)
                    }
                    frame True {
                      n253 = local read "Vname 3"() -> (w936:string)
                    }
                  }
                }
              }
            }
            frame True {
              w938 = u16 2 items=["V", "I", "VPulse", "IPulse", "Common"] ("Mode 2")
              w939 = u16 0 items=["V", "I", "VPulse", "IPulse", "Common"] ("Mode 2")
              n254 = local read "Mode 2"() -> (w940:u16)
              n255 = Equal?(x=w939, y=w940) -> (x = y?=w942:bool)
              n256 = Equal?(x=w940, y=w938) -> (x = y?=w941:bool)
              n257 = Or(x=w942, y=w941) -> (x .or. y?=w937:bool)
              n258 = case shown="True" w937 {
                tunnel: [w945 w946] -> w944
                frame False {
                  n259 = local read "Iname 2"() -> (w945:string)
                }
                frame True {
                  n260 = local read "Vname 2"() -> (w946:string)
                }
              }
            }
          }
        }
        frame True {
          w951 = u16 2 items=["V", "I", "VPulse", "IPulse", "Common"] ("Mode")
          w952 = u16 0 items=["V", "I", "VPulse", "IPulse", "Common"] ("Mode")
          n261 = local read "Mode"() -> (w950:u16)
          n262 = Equal?(x=w950, y=w952) -> (x = y?=w949:bool)
          n263 = Equal?(x=w950, y=w951) -> (x = y?=w948:bool)
          n264 = Or(x=w949, y=w948) -> (x .or. y?=w947:bool)
          n265 = case shown="True" w947 {
            tunnel: [w955 w956] -> w954
            frame False {
              n266 = local read "Iname"() -> (w955:string)
            }
            frame True {
              n267 = local read "Vname"() -> (w956:string)
            }
          }
        }
      }
      n268 = local read "error?"() -> (w577:errorcluster)
      n269 = Unbundle("Y2 axis settings") -> ("Y2 axis on/off"=w569:bool, "MINIMUM"=w582:ext, "MAXIMUM"=w581:ext, "Variable name"=w573:string, "LIN or LOG axis"=w580:string)
      n270 = local read "Var2 step settings"() -> (w592:T3)
      n271 = local read "Var1 sweep settings"() -> (w593:T4)
      n272 = local read "VISA session"() -> (w561:refnum<visa-resource-name>)
      n273 = call "Y1subvi.vi"("MAXIMUM"="MAXIMUM", "Variable name"="Y1 axis", "error in (no error)"=w577, "MINIMUM"="MINIMUM", "LIN or LOG axis"="LIN", "VISA resource name"=w561) -> ("error out"=w578:errorcluster)
      n274 = case shown="False" w569 {
        tunnel: w578 -> [w892 w899]
        tunnel: w561 -> [_ w898]
        tunnel: w582 -> [_ w897]
        tunnel: w581 -> [_ w896]
        tunnel: w573 -> [_ w895]
        tunnel: w580 -> [_ w894]
        tunnel: [w892 w893] -> w579
        frame False {
        }
        frame True {
          n275 = call "Y2subvi.vi"("MAXIMUM"=w896, "Variable name"=w895, "error in (no error)"=w899, "MINIMUM"=w897, "LIN or LOG axis"=w894, "VISA resource name"=w898) -> ("error out"=w893:errorcluster)
        }
      }
      n276 = Unbundle(w592) -> ("total points"=w591:u16)  [unwired: 4 out]
      n277 = Decrement(x=w591) -> (x-1=w551:u16)
      n278 = Unbundle(w593) -> ("start"=w559:dbl)  [unwired: 6 out]
      n279 = call "HP415xA Op-Start-Stop.vi"("error in (no error)"=w579, "function (stop:0)"=w585, "wait until finish"=TRUE, "VISA session"=w561) -> ("error out"=w584:errorcluster)  [unwired: 6 in, 1 out]
      n280 = call "HP415xA Op-Download Trace.vi"("error in (no error)"=w584, "trace (variable) name"=w590, "VISA session"=w561) -> ("error out"=w599:errorcluster, "trace"=w567:dbl[])
      n281 = call "HP415xA Op-Download Trace.vi"("error in (no error)"=w599, "trace (variable) name"="Y1 axis", "VISA session"=w561) -> ("error out"=w574:errorcluster, "trace"=w562:dbl[])
      n282 = case shown="False" w569 {
        tunnel: w574 -> [w877 w885]
        tunnel: w561 -> [_ w884]
        tunnel: w573 -> [_ w883]
        tunnel: [w877 w882] -> w563
        tunnel: w567 -> [w875 w881]
        tunnel: w562 -> [w876 w880]
        tunnel: [w874 w879] -> w570
        tunnel: [dbl[] [] ("trace") w878] -> w568
        frame False {
          n283 = Bundle("trace"=w875, "trace"=w876) -> (w874:cluster{"trace":dbl[], "trace":dbl[]})  [unwired: 1 in]
        }
        frame True {
          n284 = call "HP415xA Op-Download Trace.vi"("error in (no error)"=w885, "trace (variable) name"=w883, "VISA session"=w884) -> ("error out"=w882:errorcluster, "trace"=w878:dbl[])
          n285 = stacked-sequence {
            tunnel: w878 -> [_ w890]
            tunnel: w881 -> [w888 w889]
            tunnel: w880 -> [w887 _]
            tunnel: [w886 _] -> w879
            frame #0 {
              n286 = Bundle("trace"=w888, "trace"=w887) -> (w886:cluster{"trace":dbl[], "trace":dbl[]})  [unwired: 1 in]
            }
            frame #1 {
              n287 = Bundle("trace"=w889, "trace"=w890) -> (→"graphic display 2":cluster{"trace":dbl[], "trace":dbl[]})  [unwired: 1 in]
            }
          }
        }
      }
      "graphic display" <- w570
      n288 = case shown="True" w566 {
        tunnel: w559 -> [_ w745]
        tunnel: w562 -> [w604 w744]
        tunnel: w567 -> [w605 w742]
        tunnel: w551 -> [_ w741]
        tunnel: w561 -> [_ w737]
        tunnel: w563 -> [_ w736]
        tunnel: [w606 w735] -> w565
        tunnel: w560 -> [_ w734]
        tunnel: w560 -> [_ w727]
        tunnel: [dbl[] [] ("trace") w733] -> w564
        tunnel: w558 -> [_ w730]
        tunnel: w557 -> [_ w729]
        tunnel: w556 -> [_ w678]
        tunnel: [_ w654] -> w555
        tunnel: [_ w656] -> w554
        tunnel: w553 -> [_ w695]
        tunnel: w552 -> [_ w694]
        tunnel: w551 -> [_ _]
        tunnel: w550 -> [_ w689]
        tunnel: w549 -> [_ w607]
        frame False {
          n289 = Build Array(w605, w604) -> (w601:dbl[][])
          n290 = local read "error? 2"() -> (w606:errorcluster)
          n291 = call-poly <vilib>:"Write To Spreadsheet File.vi"("transpose? (no:F)"=TRUE ("append to file? (new file:F)"), "format (%.3f)"="%.5e", "2D data"=w601) -> ()  [unwired: 5 in, 1 out]
        }
        frame True {
          w648 = 2
          w649 = 2
          w662 = 0
          w660 = 0
          (unwired) 0.000115
          w719 = "%s"
          w669 = "\r"
          # "Vg"
          # "Dielectric"
          # "Length"
          # "Width"
          # "Sat ID"
          # "Data Values"
          # "Headers"
          n292 = Initialize Array("") -> (w708:string[])  [unwired: 1 in]
          n293 = call "HP415xA Op-Download Trace.vi"("error in (no error)"=w736, "trace (variable) name"=w734, "VISA session"=w737) -> ("error out"=w735:errorcluster, "trace"=w733:dbl[])
          n294 = for {
            N: w741 -> [w800]
            shift-right: [w817] -> w654
            shift-left: w742 -> [w813]
            tunnel: w745 -> [w819]
            tunnel: [w818] -> _ mode=indexing
            shift-right: [w814] -> w656
            shift-left: w744 -> [w816]
            tunnel: [w815] -> w743 mode=indexing
            shift-right: [w810] -> w723
            shift-left: w733 -> [w812]
            tunnel: w727 -> [_]
            tunnel: [w804] -> w725 mode=indexing
            shift-right: [w803] -> w712
            shift-left: w708 -> [w802]
            tunnel: [w800] -> _ mode=indexing
            n295 = Search 1D Array(1D array=w813, element=w819, start index (0)=1) -> (index of element=w811:i32)
            n296 = Split 1D Array(array=w812, index=w811) -> (first subarray=w808:dbl[], second subarray=w810:dbl[])
            n297 = Array Size(array=w808) -> (size(s)=w807:i32)
            n298 = Decrement(x=w807) -> (x-1=w806:i32)
            n299 = Split 1D Array(array=w813, index=w811) -> (first subarray=w818:dbl[], second subarray=w817:dbl[])
            n300 = Array Subset(array=w808, index=w806) -> (w809:dbl[])  [unwired: 1 in]
            n301 = Split 1D Array(array=w816, index=w811) -> (first subarray=w815:dbl[], second subarray=w814:dbl[])
            n302 = Number To Exponential String(number=w809) -> (E-format string=w805:string[])  [unwired: 3 in]
            n303 = Concatenate Strings(w805) -> (w804:string)
            n304 = Build Array (concatenate)("Id", w802) -> (w803:string[])
          }
          n305 = Build Array (concatenate)(w654, w743, w656) -> (w740:dbl[][])
          n306 = Transpose 2D Array(2D array=w740) -> (transposed array=w738:dbl[][])
          n307 = Array To Spreadsheet String(array=w738, 3:"%.5e" ("format string")) -> (spreadsheet string=w728:string)  [unwired: 1 in]
          n308 = local read "Temp (K)"() -> (w646:dbl)
          n309 = Number To Exponential String(number=w646) -> (E-format string=w645:string)  [unwired: 3 in]
          n310 = local read "Vt"() -> (w639:dbl)
          n311 = Build Array("Sample Temp (K):", w645) -> (w644:string[])
          n312 = Build Array("Vg", "Id") -> (w713:string[])
          n313 = Array Size(array=w723) -> (size(s)=w724:i32)
          n314 = Fract/Exp String To Number(string="") -> (number=w629:dbl)  [unwired: 3 in, 1 out]
          n315 = Reshape Array(w644, 1 ("start index (0)")) -> (w641:string[])
          n316 = Decrement(x=w724) -> (x-1=w722:i32)
          n317 = Array Subset(array=w723, index=w722) -> (w721:dbl[])  [unwired: 1 in]
          n318 = Insert Into Array(array=w713, index=2, new element=w712) -> (w711:string[])
          n319 = Number To Exponential String(number=w721) -> (E-format string=w717:string[])  [unwired: 3 in]
          n320 = Array To Spreadsheet String(array=w641, 3:"%s") -> (spreadsheet string=w640:string)  [unwired: 1 in]
          n321 = Build Array("Mobility-Sat (cm^2/Vs):", "Mobility-Lin (cm^2/Vs):", "On/Off I-Sat:", "Off I-Sat (A):", "Vt-Sat (V):", "STS-Sat (V/decade):", "Trap Density-VT (Traps/Vcm^2):", "Trap Density-STS (Traps/Vcm^2):") -> (w676:string[])
          n322 = Array To Spreadsheet String(array=w711, 3:w719) -> (spreadsheet string=w718:string)  [unwired: 1 in]
          n323 = Concatenate Strings(w717) -> (w716:string)
          n324 = Build Array (concatenate)("Vd=", w725, w716) -> (w720:string[])
          n325 = Array To Spreadsheet String(array=w720, 3:w719) -> (spreadsheet string=w726:string)  [unwired: 1 in]
          n326 = local read "Input Path"() -> (w609:path)
          n327 = Fract/Exp String To Number(string=w695) -> (number=w666:dbl)  [unwired: 3 in, 1 out]
          n328 = Fract/Exp String To Number(string=w694) -> (number=w667:dbl)  [unwired: 3 in, 1 out]
          n329 = Fract/Exp String To Number(string=w607) -> ()  [unwired: 3 in, 2 out]
          n330 = Initialize Array(0) -> (w692:i32[])  [unwired: 1 in]
          n331 = Initialize Array(w660, w649) -> (w661:i32[])
          n332 = Initialize Array(w660, w649) -> (w659:i32[])
          n333 = Array Size(array=w654) -> (size(s)=w682:i32)
          n334 = for {
            N: w682 -> [w748]
            shift-right: [w751] -> w681
            shift-left: w656 -> [w752]
            i -> [w747]
            n335 = Subtract(x=w748, y=w747) -> (x-y=w746:i32)
            n336 = Index Array(array=w752, index=w746) -> (element=w749:dbl)
            n337 = Greater Or Equal To 0?(x=w749) -> (x >= 0?=w750:bool)
            n338 = case shown="True" w750 {
              tunnel: w752 -> [w753 w756]
              tunnel: w746 -> [_ w754]
              tunnel: [w753 w755] -> w751
              frame False {
              }
              frame True {
                n339 = Delete From Array(array=w756, index=w754) -> (array with subset deleted=w755:dbl[])  [unwired: 1 in, 1 out]
              }
            }
          }
          n340 = Initialize Array(w660) -> (w664:i32[])  [unwired: 1 in]
          n341 = local read "NumPts"() -> (w608:dbl)
          n342 = Subtract(x=w682, y=w608) -> (x-y=w693:dbl)
          n343 = for {
            N: w693 -> [_]
            shift-right: [w794] -> _
            shift-left: w654 -> [w794]
            shift-right: [w795] -> _
            shift-left: w656 -> [w795]
            shift-right: [w799] -> w698
            shift-left: w692 -> [w798]
            shift-right: [w797] -> w696
            shift-left: w664 -> [w796]
            tunnel: w608 -> [w789]
            shift-right: [w785] -> w663
            shift-left: w661 -> [w788]
            shift-right: [w782] -> w652
            shift-left: w659 -> [w783]
            i -> [w786]
            n344 = Array Subset(array=w794, index=w786, length=w789) -> (w784:dbl[])
            n345 = Array Subset(array=w795, index=w786, length=w789) -> (w793:dbl[])
            n346 = Absolute Value(x=w793) -> (abs(x)=w792:dbl[])
            n347 = Build Array (concatenate)(w783, w784) -> (w782:dbl[])
            n348 = Square Root(x=w792) -> (sqrt(x)=w787:dbl[])
            n349 = call <vilib>:"Linear Fit.vi"("Y"=w787, "X"=w784) -> ("Best Linear Fit"=w791:dbl[], "slope"=w781:dbl, "intercept"=w779:dbl)  [unwired: 9 in, 2 out]
            n350 = Insert Into Array(array=w788, index=w786, new element=w787) -> (w785:i32[])
            n351 = call <vilib>:"Goodness of Fit.vi"("Best Fit"=w791, "Y"=w787) -> ("R-square"=w790:dbl)  [unwired: 6 in, 3 out]
            n352 = Negate(x=w781) -> (-x=w780:dbl)
            n353 = Divide(x=w780, y=w779) -> ()  [unwired: 1 out]
            n354 = Build Array (concatenate)(w796, w790) -> (w797:dbl[])
            n355 = Build Array (concatenate)(w798, w781) -> (w799:dbl[])
          }
          n356 = Array Max & Min(array=w681) -> (max value=w679:dbl, min value=w680:dbl)  [unwired: 2 out]
          n357 = Divide(x=w680, y=w679) -> (x/y=w631:dbl)
          n358 = Absolute Value(x=w656) -> (abs(x)=w658:dbl[])
          n359 = Square Root(x=w658) -> (sqrt(x)=w657:dbl[])
          n360 = Initialize Array(w662, w648) -> (w651:i32[])
          n361 = local write "On/Off Current"(w631) -> ()
          n362 = Initialize Array(w662, w648) -> (w668:i32[])
          n363 = for {
            N: 20 -> [_]
            shift-right: [w777] -> _
            shift-left: w696 -> [w778]
            shift-right: [w769] -> _
            shift-left: w698 -> [w767]
            shift-right: [w768] -> w699
            shift-left: w668 -> [w776]
            shift-right: [w775] -> w690
            shift-left: w668 -> [w774]
            shift-right: [w765] -> _
            shift-left: w663 -> [w766]
            shift-right: [w764] -> w619
            shift-left: w651 -> [w772]
            shift-right: [w757] -> _
            shift-left: w652 -> [w759]
            shift-right: [w761] -> w618
            shift-left: w651 -> [w760]
            w763 = 1
            n364 = Array Max & Min(array=w778) -> (max value=w773:dbl, max index (indices)=w758:i32)  [unwired: 2 out]
            n365 = Array Subset(array=w759, index=w758, length=w763) -> (w762:dbl[])
            n366 = Array Subset(array=w766, index=w758, length=w763) -> (w771:i32[])
            n367 = Array Subset(array=w767, index=w758, length=w763) -> (w770:dbl[])
            n368 = Build Array (concatenate)(w776, w770) -> (w768:dbl[])
            n369 = Delete From Array(array=w778, index=w758) -> (array with subset deleted=w777:dbl[])  [unwired: 1 in, 1 out]
            n370 = Build Array (concatenate)(w760, w762) -> (w761:dbl[])
            n371 = Build Array (concatenate)(w774, w773) -> (w775:dbl[])
            n372 = Build Array (concatenate)(w772, w771) -> (w764:i32[])
            n373 = Delete From Array(array=w766, index=w758) -> (array with subset deleted=w765:i32[])  [unwired: 1 in, 1 out]
            n374 = Delete From Array(array=w759, index=w758) -> (array with subset deleted=w757:dbl[])  [unwired: 1 in, 1 out]
            n375 = Delete From Array(array=w767, index=w758) -> (array with subset deleted=w769:dbl[])  [unwired: 1 in, 1 out]
          }
          "Max R" <- w690
          n376 = Bundle("trace"=w654, w657) -> (w655:cluster{"trace":dbl[], dbl[]})  [unwired: 1 in]
          n377 = local read "Vt"() -> (w638:dbl)
          n378 = Absolute Value(x=w638) -> (abs(x)=w637:dbl)
          n379 = Fract/Exp String To Number(string=w689) -> (number=w684:dbl)  [unwired: 3 in, 1 out]
          n380 = Array Max & Min(array=w699) -> (min value=w650:dbl, min index (indices)=w620:i32)  [unwired: 2 out]
          n381 = Multiply(x=w620, y=w608) -> (x*y=w622:dbl)
          n382 = Array Subset(array=w618, index=w622, length=w608) -> (w623:dbl[])
          n383 = Array Subset(array=w619, index=w622, length=w608) -> (w624:i32[])
          n384 = call <vilib>:"Linear Fit.vi"("Y"=w624, "X"=w623) -> ("slope"=w627:dbl, "intercept"=w625:dbl)  [unwired: 9 in, 3 out]
          n385 = Negate(x=w625) -> (-x=w626:dbl)
          n386 = Divide(x=w626, y=w627) -> (x/y=w621:dbl)
          n387 = Bundle(w623, w624) -> (w617:cluster{dbl[], i32[]})  [unwired: 1 in]
          n388 = local write "Vt"(w621) -> ()
          n389 = Build Array(w655, w617) -> (→"XY Graph":cluster{"trace":dbl[], dbl[]}[])
          n390 = Square(x=w650) -> (x^2=w700:dbl)
          n391 = Multiply(x=2, y=w700) -> (x*y=w701:dbl)
          n392 = Multiply(x=3.9, y=8.854e-12) -> (x*y=w686:dbl)
          n393 = Multiply(x=w667, y=w701) -> (x*y=w702:dbl)
          n394 = Multiply(x=w684, y=1e-09) -> (x*y=w683:dbl)
          n395 = Divide(x=w686, y=w683) -> (x/y=w636:dbl)
          n396 = Multiply(x=w637, y=w636) -> (x*y=w635:dbl)
          n397 = Divide(x=w635, y=1.602e-19) -> (x/y=w632:dbl)
          n398 = Multiply(x=w666, y=w636) -> (x*y=w703:dbl)
          n399 = local write "Trap Density-VT"(w632) -> ()
          n400 = Divide(x=w702, y=w703) -> (x/y=w705:dbl)
          n401 = Multiply(x=w705, y=10000) -> (x*y=w633:dbl)
          n402 = Build Array(w633, w631, w639, w629, w632, w629) -> (w675:dbl[])
          n403 = Number To Exponential String(number=w675) -> (E-format string=w674:string[])  [unwired: 3 in]
          n404 = Build Array(w676, w674) -> (w673:string[][])
          n405 = Transpose 2D Array(2D array=w673) -> (transposed array=w672:string[][])
          n406 = Array To Spreadsheet String(array=w672, 3:"%s") -> (spreadsheet string=w670:string)  [unwired: 1 in]
          n407 = Concatenate Strings(w730, w669, w729, w669, w678, w640, w669, w670, w669, w726, w718, w728, "\r") -> (w732:string)
          n408 = call <vilib>:"Write Characters To File.vi"("append to file? (new file:F)"=TRUE, "character string"=w732, "file path (dialog if empty)"=w609) -> ("new file path (Not A Path if cancelled)"=w628:path)  [unwired: 2 in]
          n409 = local write "Output Path"(w628) -> ()
          n410 = local write "Mobility"(w633) -> ()
        }
      }
      n411 = case shown="True" w569 {
        tunnel: w551 -> [_ w826]
        tunnel: w566 -> [_ w827]
        tunnel: w567 -> [_ w825]
        tunnel: w559 -> [_ w824]
        tunnel: w568 -> [_ w823]
        tunnel: w564 -> [_ w822]
        tunnel: w560 -> [_ w821]
        frame False {
        }
        frame True {
          n412 = case shown="True" w827 {
            tunnel: w826 -> [_ w843]
            tunnel: w825 -> [w831 w858]
            tunnel: w824 -> [_ w857]
            tunnel: w823 -> [w832 w856]
            tunnel: w822 -> [_ w855]
            tunnel: w821 -> [_ w838]
            frame False {
              n413 = Build Array(w831, w832) -> (w830:dbl[][])
              n414 = call-poly <vilib>:"Write To Spreadsheet File.vi"("transpose? (no:F)"=TRUE, "format (%.3f)"="%.5e", "2D data"=w830) -> ()  [unwired: 5 in, 1 out]
            }
            frame True {
              n415 = for {
                N: w843 -> [_]
                shift-right: [w869] -> w854
                shift-left: w858 -> [w870]
                tunnel: w857 -> [w872]
                tunnel: [w868] -> _ mode=indexing
                shift-right: [w865] -> w852
                shift-left: w856 -> [w867]
                tunnel: [w866] -> w853 mode=indexing
                shift-right: [w862] -> w847
                shift-left: w855 -> [w863]
                tunnel: [w859] -> w844 mode=indexing
                n416 = Search 1D Array(1D array=w870, element=w872, start index (0)=1) -> (index of element=w864:i32)
                n417 = Split 1D Array(array=w870, index=w864) -> (first subarray=w868:dbl[], second subarray=w869:dbl[])
                n418 = Split 1D Array(array=w867, index=w864) -> (first subarray=w866:dbl[], second subarray=w865:dbl[])
                n419 = Split 1D Array(array=w863, index=w864) -> (first subarray=w860:dbl[], second subarray=w862:dbl[])
                n420 = Index Array(array=w860, index=1) -> (element=w859:dbl)
              }
              n421 = Build Array (concatenate)(w854, w853, w852) -> (w851:dbl[][])
              n422 = Index Array(array=w847, index=1) -> (element=w845:dbl)
              n423 = Transpose 2D Array(2D array=w851) -> (transposed array=w850:dbl[][])
              n424 = Insert Into Array(array=w844, index=w843, new element=w845) -> (w842:dbl[])
              n425 = Array To Spreadsheet String(delimiter (Tab)=",", array=w842, 3:"%.5e" ("format string")) -> (spreadsheet string=w836:string)
              n426 = Array To Spreadsheet String(delimiter (Tab)=",", array=w850, 3:"%.5e" ("format string")) -> (spreadsheet string=w834:string)
              n427 = Concatenate Strings(w838, "," ("string")) -> (w837:string)
              n428 = Concatenate Strings(w837, w836) -> (w835:string)
              n429 = Concatenate Strings(w835, w834) -> (w833:string)
              n430 = call <vilib>:"Write Characters To File.vi"("character string"=w833) -> ()  [unwired: 4 in, 1 out]
            }
          }
        }
      }
      n431 = call "HP415xA Sys-Error Query.vi"("VISA session"=w561, "error in (no error)"=w565) -> ("error out"=w597:errorcluster)  [unwired: 2 in, 1 out]
      n432 = call "HP415xA  Close.vi"("error in (no error)"=w597, "VISA session"=w561) -> ("error out"=w598:errorcluster)
      n433 = local write "error?"(w598) -> ()
    }
    frame #6 {
      n434 = flat-sequence {
        frame #0 {
          n435 = local read "Output Path"() -> (w989:path)
          n436 = local read "Sample Properties:"() -> (w985:T1)
          n437 = local read "Temp (K)"() -> (w976:dbl)
          n438 = call "sub_thresh_swing_subvi.vi"("Path"=w989) -> ("Sub Threshold Swing"=w975:dbl)  [unwired: 10 in, 4 out]
          n439 = Unbundle By Name(w985) -> ("SiO2 Thickness"=w978:string)
          n440 = Equal To 0?(x=w976) -> (x = 0?=w988:bool)
          n441 = local write "STS"(w975) -> ()
          n442 = case shown="True" w988 {
            tunnel: [w990 290] -> w987
            tunnel: w976 -> [w990 _]
            frame False {
            }
            frame True {
            }
          }
          n443 = Fract/Exp String To Number(string=w978) -> (number=w980:dbl)  [unwired: 3 in, 1 out]
          n444 = Multiply(x=3.9, y=8.854e-12) -> (x*y=w984:dbl)
          n445 = Multiply(x=w980, y=1e-09) -> (x*y=w981:dbl)
          n446 = Divide(x=w984, y=w981) -> (x/y=w977:dbl)
          n447 = call "Trap Density_STS.vi"("Temp (T) [K]"=w987, "S.T.S. (S)"=w975, "Dielectric"=w977) -> ("Trap Density (N)"=w986:dbl)  [unwired: 8 in]
          n448 = local write "Trap Density-STS"(w986) -> ()
        }
        frame #1 {
          n449 = local read "Output Path"() -> (w992:path)
          n450 = call-poly <vilib>:"Read From Spreadsheet File.vi"("file path (dialog if empty)"=w992) -> ("all rows"=w999:string[][])  [unwired: 6 in, 4 out]
          n451 = Array Subset(array=w999, index (col)=0, length (col)=1) -> (w1007:string[][])  [unwired: 2 in]
          n452 = Reshape Array(w1007, 100) -> (w1004:string[])
          n453 = Search 1D Array(1D array=w1004, element="S.T.S. (V/decade):") -> (index of element=w1002:i32)  [unwired: 1 in]
          n454 = Search 1D Array(1D array=w1004, element="Trap Density-STS (Traps/Vcm^2):") -> (index of element=w996:i32)  [unwired: 1 in]
          n455 = local read "Trap Density-STS"() -> (w995:dbl)
          n456 = local read "STS"() -> (w1003:dbl)
          n457 = Number To Exponential String(number=w1003) -> (E-format string=w1000:string)  [unwired: 3 in]
          n458 = Replace Array Subset(array=w999, new element=w1000, index (row)=w1002, index (col)=1) -> (w998:string[][])
          n459 = Number To Exponential String(number=w995) -> (E-format string=w994:string)  [unwired: 3 in]
          n460 = Replace Array Subset(array=w998, new element=w994, index (row)=w996, index (col)=1) -> (w993:string[][])
          "Array" <- w993
          n461 = call-poly <vilib>:"Write To Spreadsheet File.vi"("2D data"=w993, "file path (dialog if empty)"=w992) -> ()  [unwired: 6 in, 1 out]
        }
      }
    }
  }
